vi "main_scan.vi"() -> ()   [LabVIEW 2009]
uses:
  <vilib>/userDefined/High Color/IMAQdx.ctl
  <vilib>/vision/Image Controls.llb/IMAQ Image.ctl
  global_stage_initialised.vi
  <vilib>/vision/driver/IMAQdx.llb/IMAQdx Buffer Number Mode.ctl
  <vilib>/Utility/file.llb/Write To Spreadsheet File (DBL).vi
  <vilib>/vision/driver/NI_Vision_Acquisition_Software.lvlib
  C:/Program Files/National Instruments/LabVIEW 2009/resource/objmgr/imaqdx.rc
panel:
  in  "Max. Spannungsdifferenz":dbl=150.0
  out "Geschätzte Messzeit":string="00:00"
  out "Start time [ms]":timestamp
  out "2D-Intensitätsverteilung (MCP)":dbl[][](graph)
  in  "# Photosignale":i32
  in  "Achs-ID":i32
  in  "Spannungskanal":refnum<k21>
  out "x-U-Scan läuft":bool
  out "Spannungsscan läuft":bool
  out "LAPD Spannung (V)":dbl format="%#.3g"
  out "Summierte Helligkeit (a.u.)":u64
  out "# Messschritte":i32
  out "Aktueller Messschritt":i32
  in  "LAPD-Daten speichern":bool
  in  "Summierte Helligkeit speichern":bool
  in  "Einzelbilder speichern":bool
  in  "Gemittelte Bilder speichern":bool
  in  "# Bilder/Messschritt":i32=1
  in  "SN von Rotationsbühne":i32=83831982
  in  "Wellenplatte [°]":refnum<k7>(container)
  out "Wellenplatte":bool
  in  "Waveplate ON/OFF":bool
  in  "Registerkarte":T1(tab)=enum."x-U-Scan"
  out "Aktuelle xyz-Position [mm]":dbl[](array[numeric]) format="%.5g"
  in  "Rasterweite [µm]":dbl[](array[numeric])
  in  "# Rasterschritte":i32[](array[numeric])=[1, 1, 1] min=1 step=1
  in  "Rasterung ON/OFF":bool
  out "Start xyz-Position [mm]":dbl[](array[numeric]) format="%.5g"
  in  "Rasterart":T2(ring)=enum."2D-Scan(xy)"
  out "Rasterschritt [µm]":dbl[](array[numeric])
  out "2D-Intensitätsverteilung (LAPD)":dbl[][](graph)
  out "Spannungsstart [V]":dbl[](array[numeric])
  out "TIP/SUP":string[](array[string])=["Tip", "Suppressor"]
  out "Spannungsschritt [V]":dbl[](array[numeric]) format="%.1g"
  out "Aktuelle Spannung [V]":dbl[](array[numeric]) format="%.1f"
  in  "# Spannungsschritte":i32[](array[numeric])
  in  "Spannungsweite [V]":dbl[](array[numeric])
  in  "Spannungsscan ON/OFF":bool
  out "x-U-Scan Spannungsstart [V]":dbl
  out "x-U-Scan Spannungsschritt [V]":dbl
  out "x-U-Scan aktuelle Spannung [V]":dbl
  in  "# x-U-Scan Spannungsschritte":i32
  in  "x-U-Scan Spannungsweite [V]":dbl
  in  "Raum-Koordinate":enum16{"x-Achse", "y-Achse", "z-Achse"}(ring)
  in  "Spannungs-Koordinate":enum16{"Tip-Spannung", "Suppressor-Spannung"}(ring)=2
  in  "x-U-Scan ON/OFF":bool
  in  "x-U-Scan Rasterweite [µm]":dbl
  in  "# x-U-Scan Rasterschritte":i32
  out "x-U-Scan Startposition [mm]":dbl format="%.4g"
  out "x-U-Scan aktuelle Position [mm]":dbl format="%.4g"
  out "x-U-Scan Rasterschritt [µm]":dbl
  in  "Sequenz Ordner":string="Referenzbilder"
  in  "Sequenzaufnahme ON":bool
  in  "MCP-Spannung [V]":dbl=1400.0
  in  "P-Schirm-Spannung [V]":dbl=4400.0
  in  "Proben-ID":string="140528_06"
  out "Messlogbuch":path
  out "Gemitteltes Bild":u64[][](array[numeric])
  in  "Polarisation [°]":dbl=90.0
  out "Current y step":i32
  out "Current x step":i32
  out "Current z step":i32
  out "Scanschleifenzähler":i32
  out "Kameraschleifenzähler":i32
  out "Steuerschleifenzähler":i32
  out "Bühne":bool
  in  "HV ON/OFF":bool
  out "HV-Steuerung":bool
  in  "Suppressor-Spannung [V]":dbl min=0.0 max=1000.0 step=1.0 format="%.1p"
  in  "Tip-Spannung [V]":dbl min=0.0 max=800.0 step=1.0 format="%.1p"
  in  "Leistung (iK) [mW]":dbl format="%.1g"
  in  "LAPD-Kanal (Meilhaus)":u32=1 max=31
  out "Save folder":string
  out "Buffer Number":u64
  out "ROI table":string[](array[string])=["Breite [px]", "Höhe [px]", "X-Offset [px]", "Y-Offset [px]"]
  in  "Vollbild":bool
  out "Frame Rate (FPS)":dbl format="%#_3g"
  in  "Buffer Interval":u32=1
  out "Ereignis: FrameDone?":refnum<event-registration>
  out "Image Display":T3(plugin-control)
  in  "ROI":i32[](array[numeric])=[640, 480, 0, 0]
  in  "Shutter time (ms)":u16(ring)=3 items=["1000", "500", "200", "100", "50", "20", "10"]
  out "Buffer Overrun":bool
  out "Image Memory":T3
  out "Kamera":bool
  in  "Kamera ON/OFF":bool
  in  "Detektionskamera":T4="cam0"
  out "Day folder":string
  in  "Root folder":string="E:\\GIPES\\Messungen\\"
  out "z-Achse":i32=3
  out "y-Achse":i32=2
  out "x-Achse":i32=1
  out "Event: Rasterung gestartet?":refnum<user-event>
  out "Fehler (Ausgang)":errorcluster
  in  "Programm beenden":bool
  out "Rasterung läuft":bool
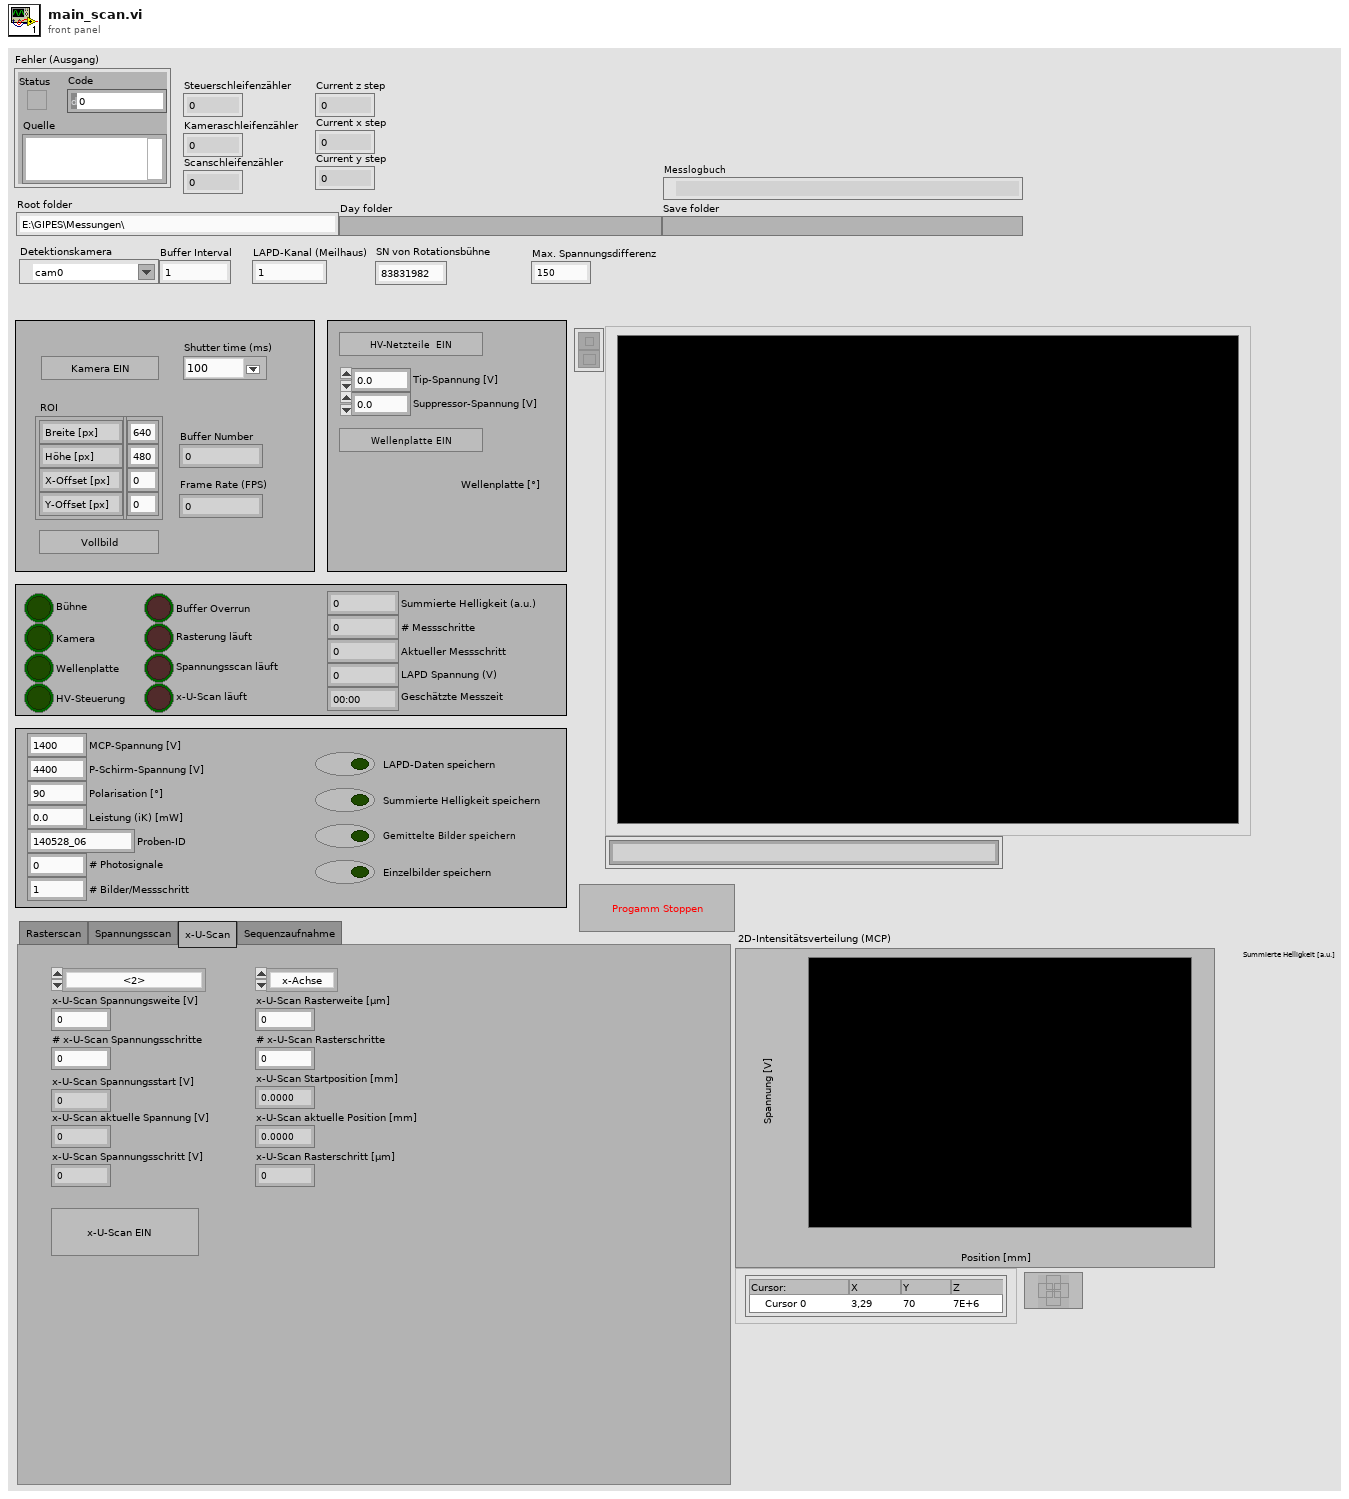
[diagram p1: front panel]
types:
  T1 = enum32{"Rasterscan", "Spannungsscan", "x-U-Scan", "Sequenzaufnahme"}
  T2 = enum16{"Linescan(x)", "Linescan(z)", "2D-Scan(xy)", "2D-Scan(yz)"}
  T3 = typedef "IMAQ Image.ctl" = refnum<image>
  T4 = typedef "IMAQdx.ctl" = refnum<k21>
  T5 = enum32{"Bad", "Idle", "Run top level", "Running"}
  T6 = typedef "NI_Vision_Acquisition_Software.lvlib/IMAQdx Buffer Number Mode.ctl" = enum32{"Next", "Last", "Buffer Number"}
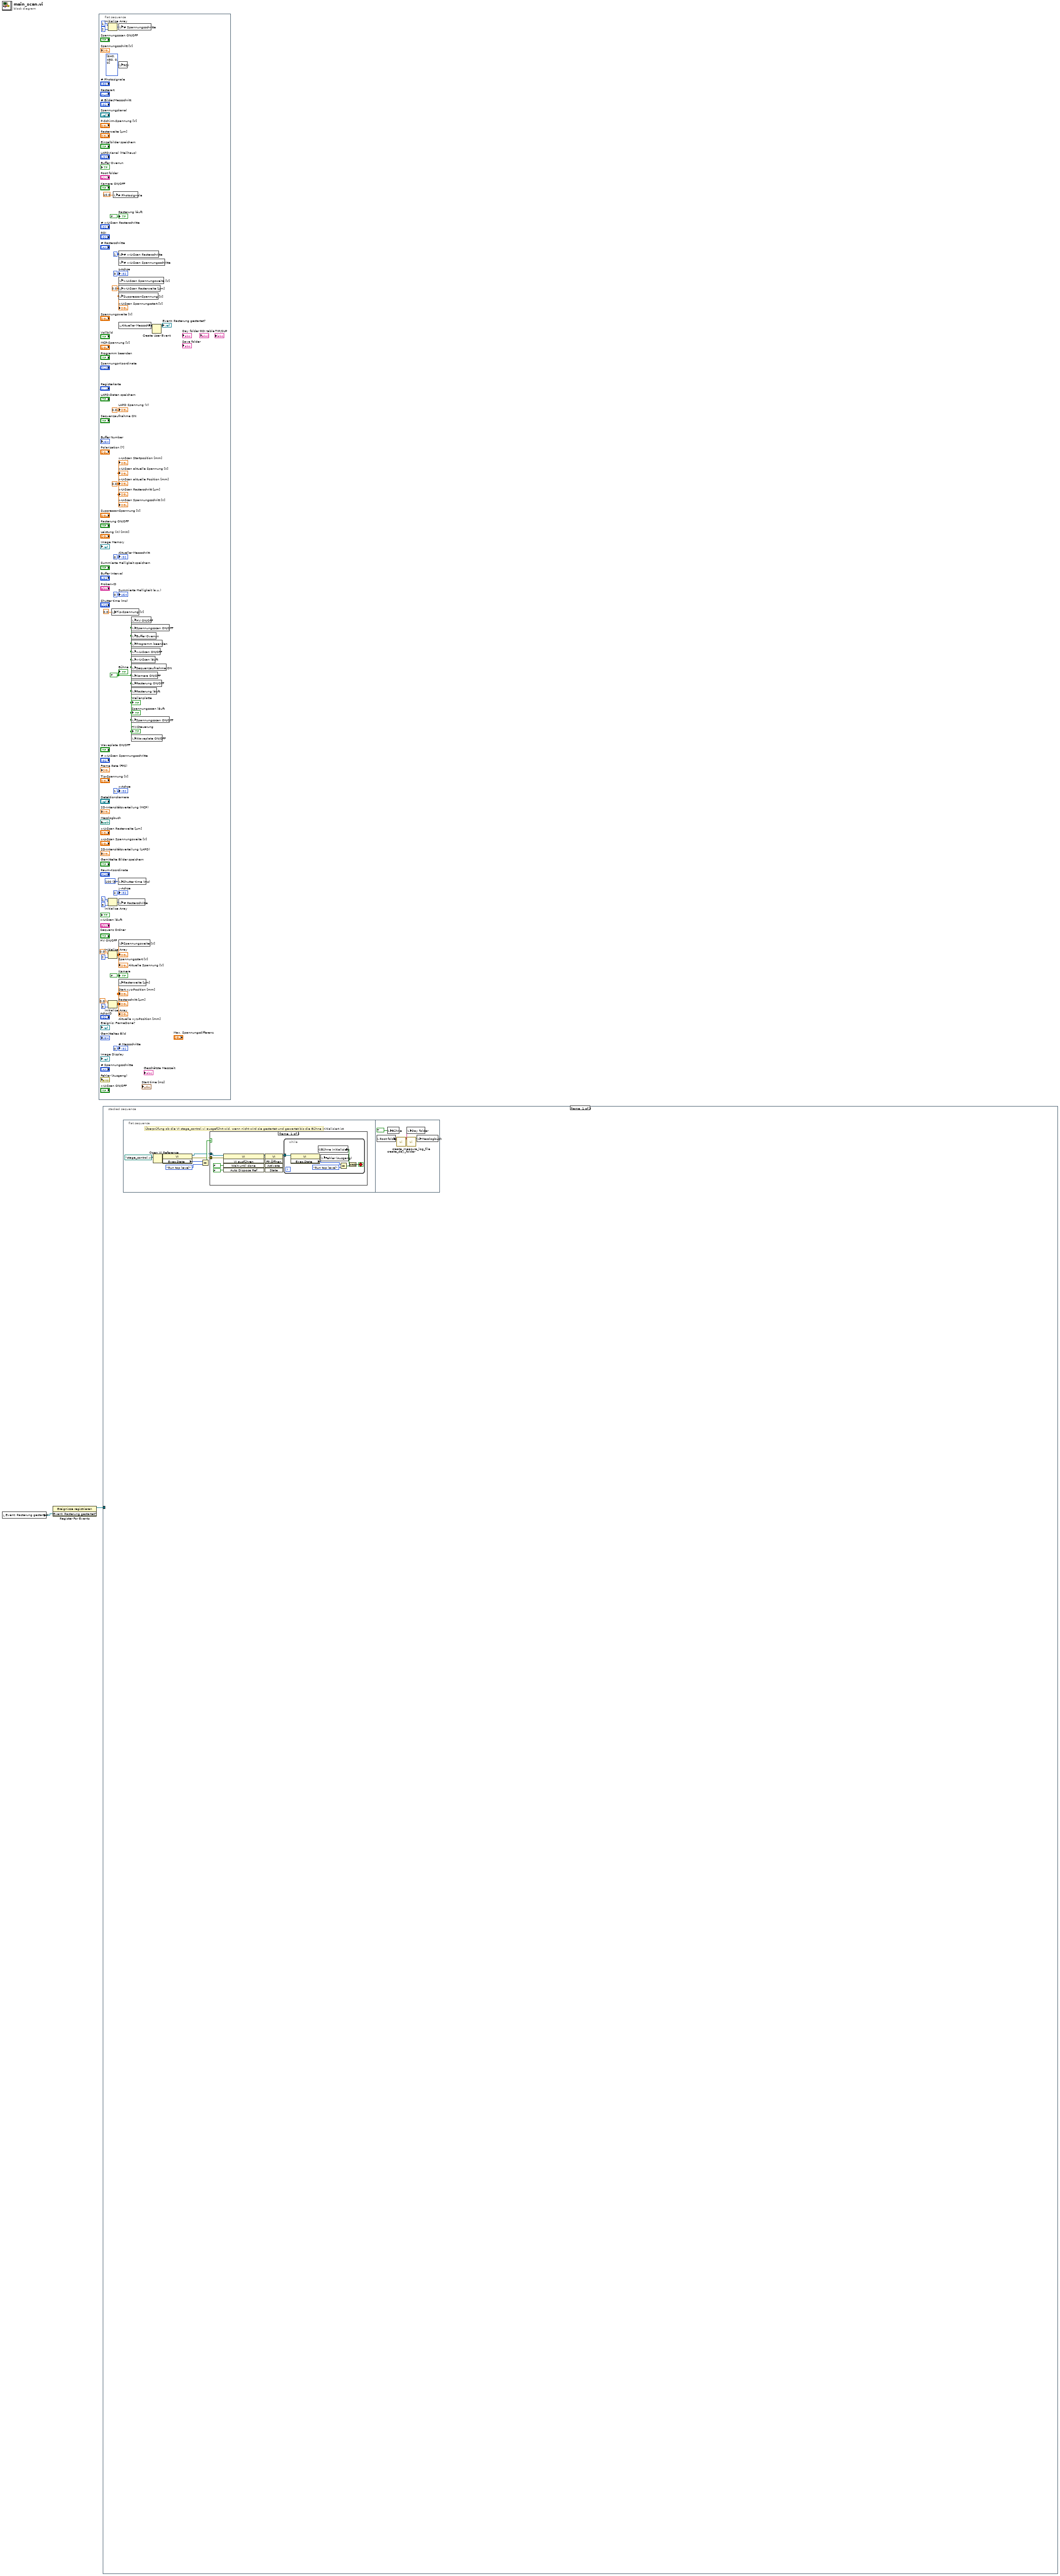
[diagram p0: block diagram]
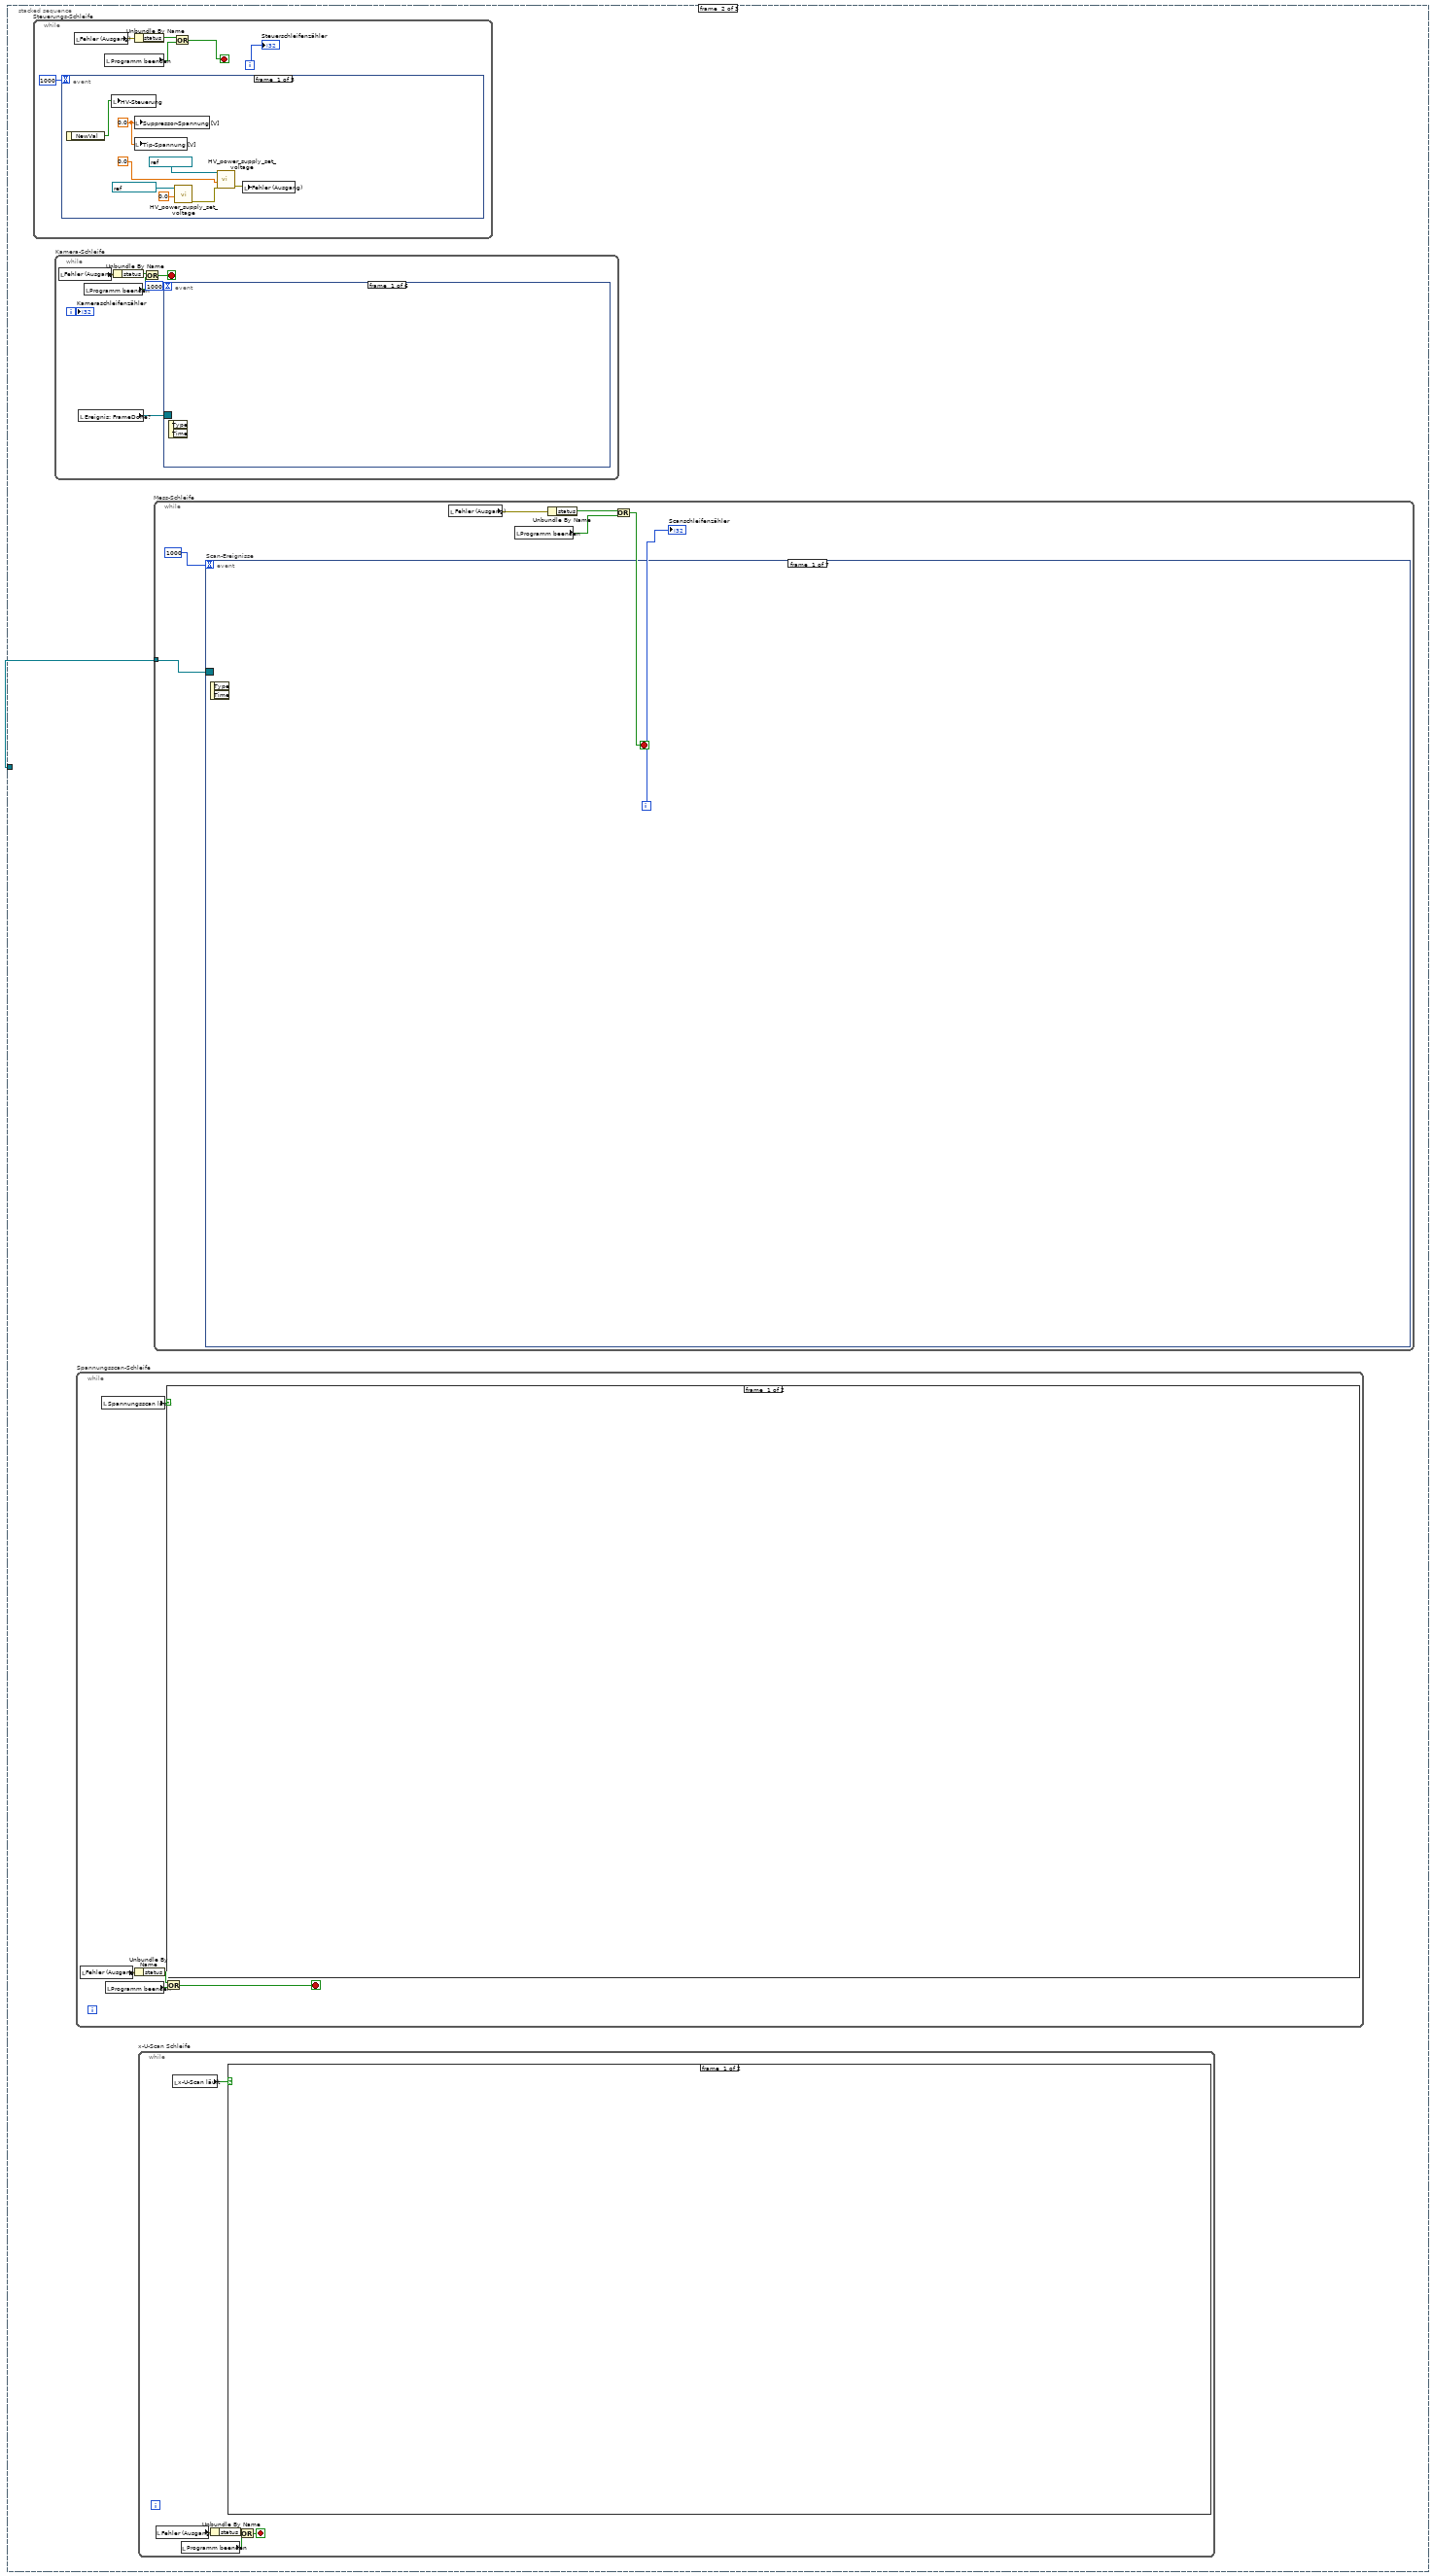
[diagram p3: hidden frame]
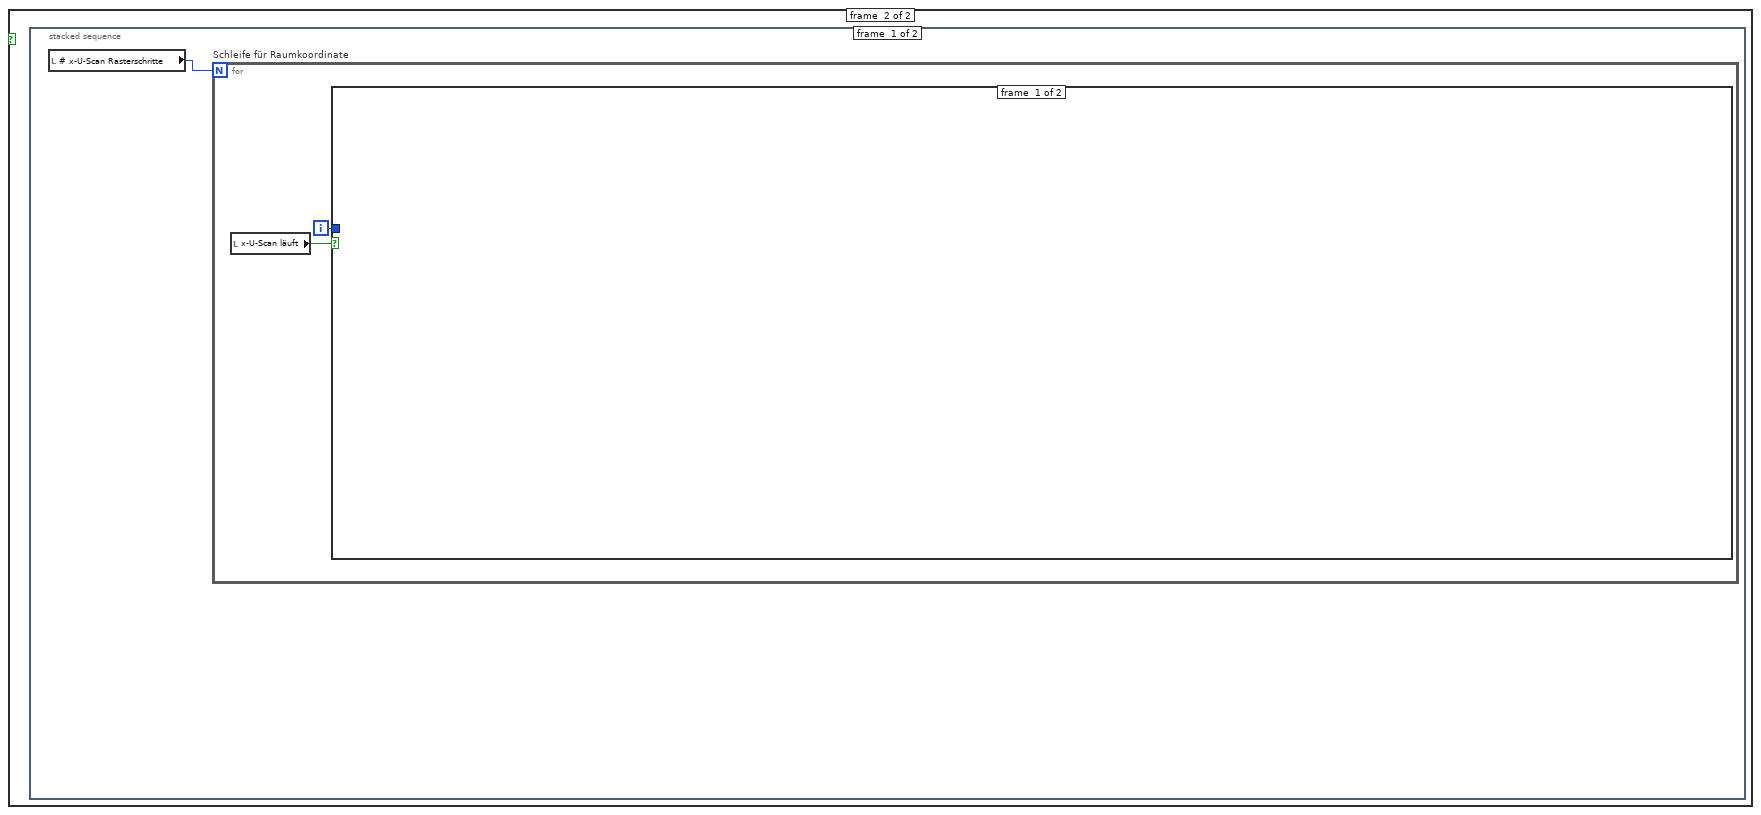
[diagram p4: hidden frame]
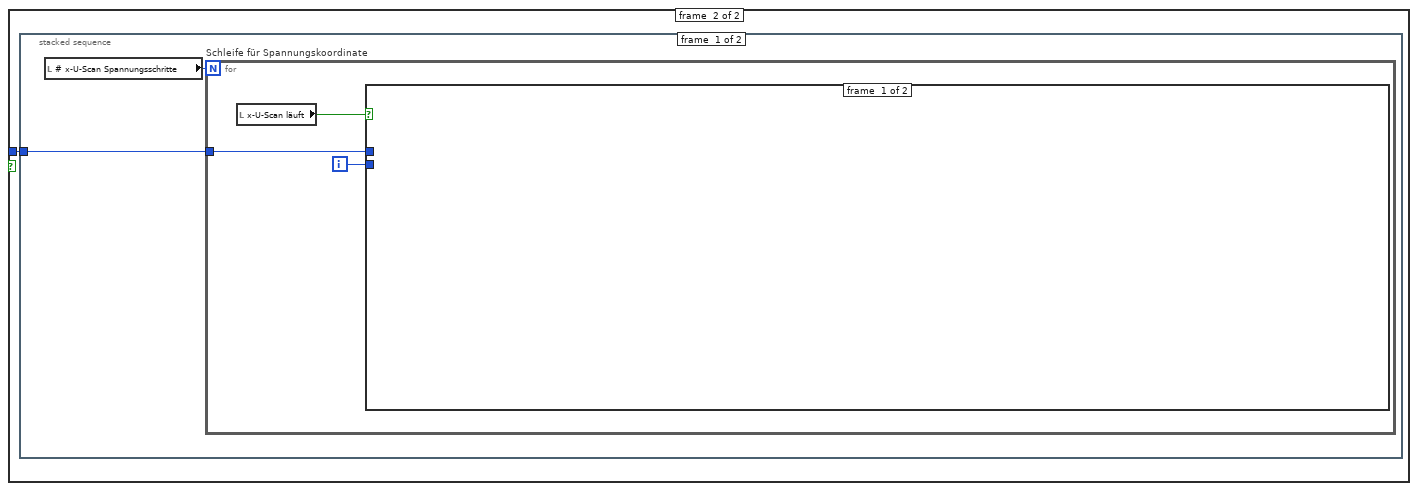
[diagram p5: hidden frame]
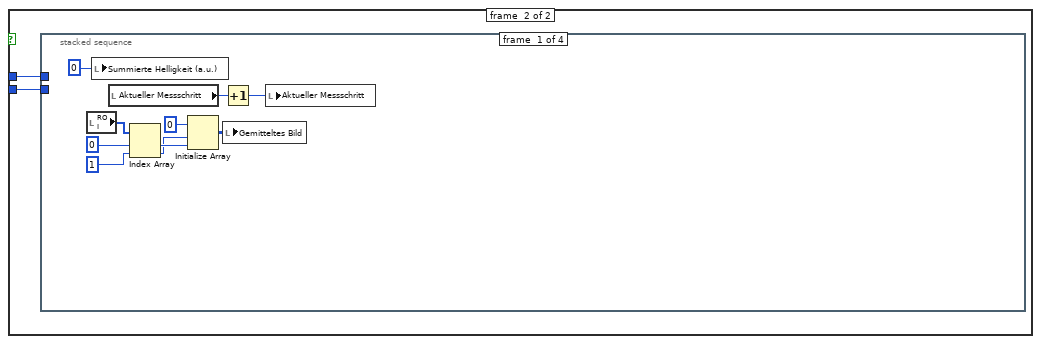
[diagram p6: hidden frame]
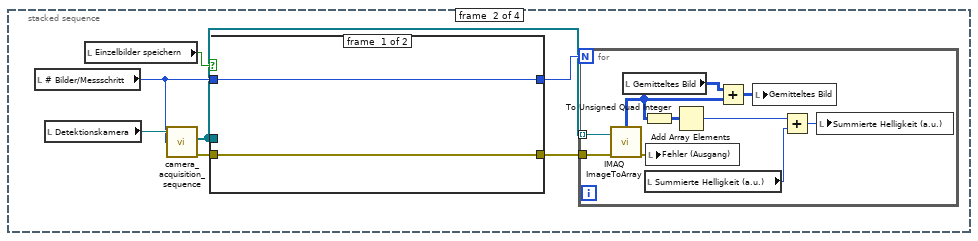
[diagram p7: hidden frame]
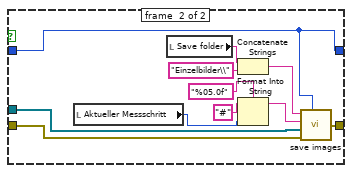
[diagram p8: hidden frame]
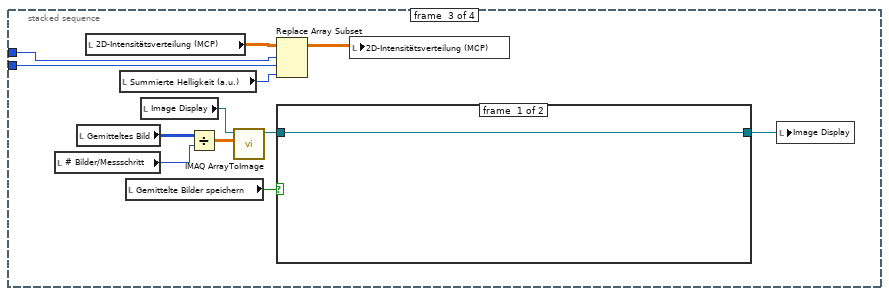
[diagram p9: hidden frame]
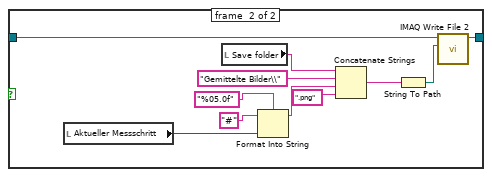
[diagram p10: hidden frame]
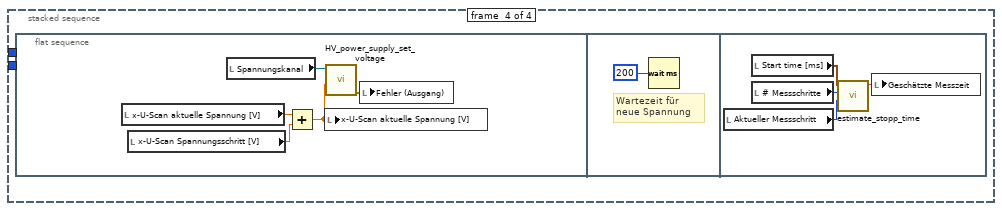
[diagram p11: hidden frame]
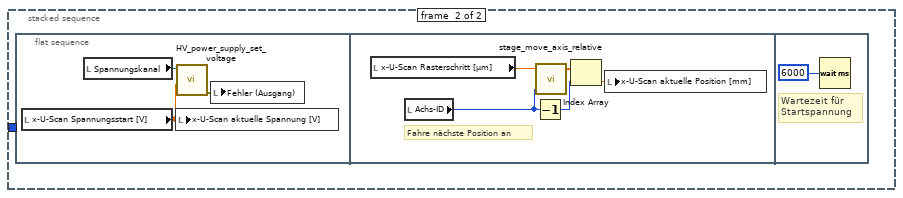
[diagram p12: hidden frame]
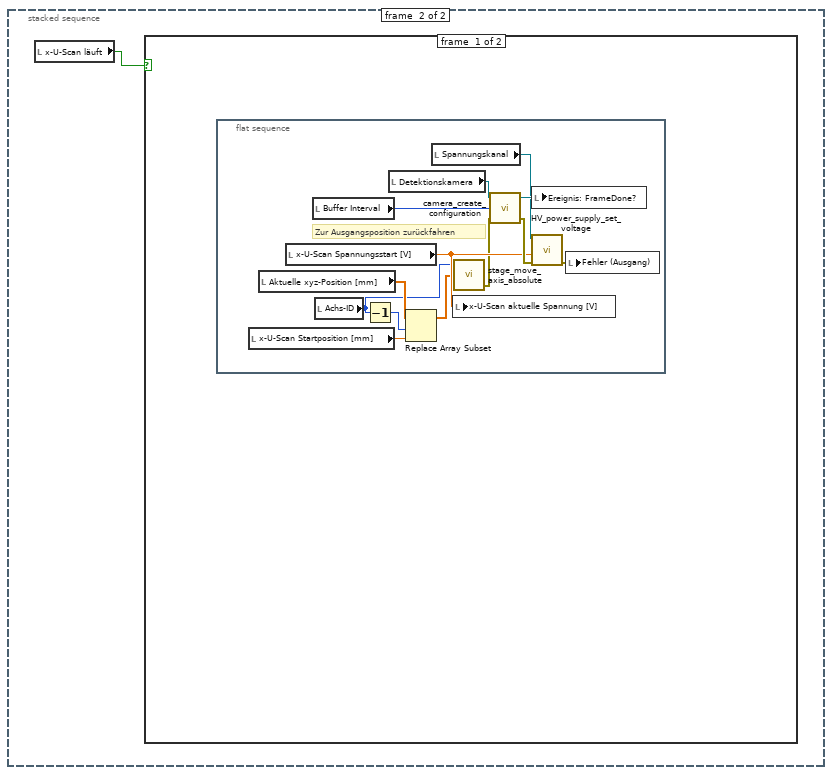
[diagram p13: hidden frame]
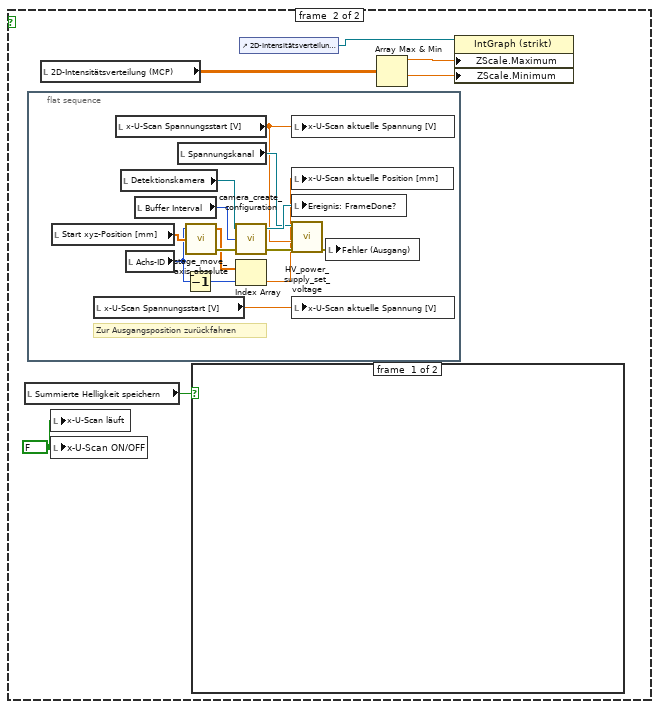
[diagram p14: hidden frame]
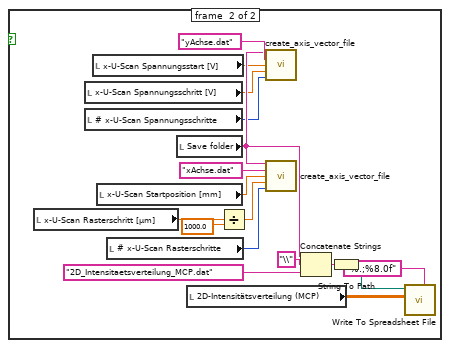
[diagram p15: hidden frame]
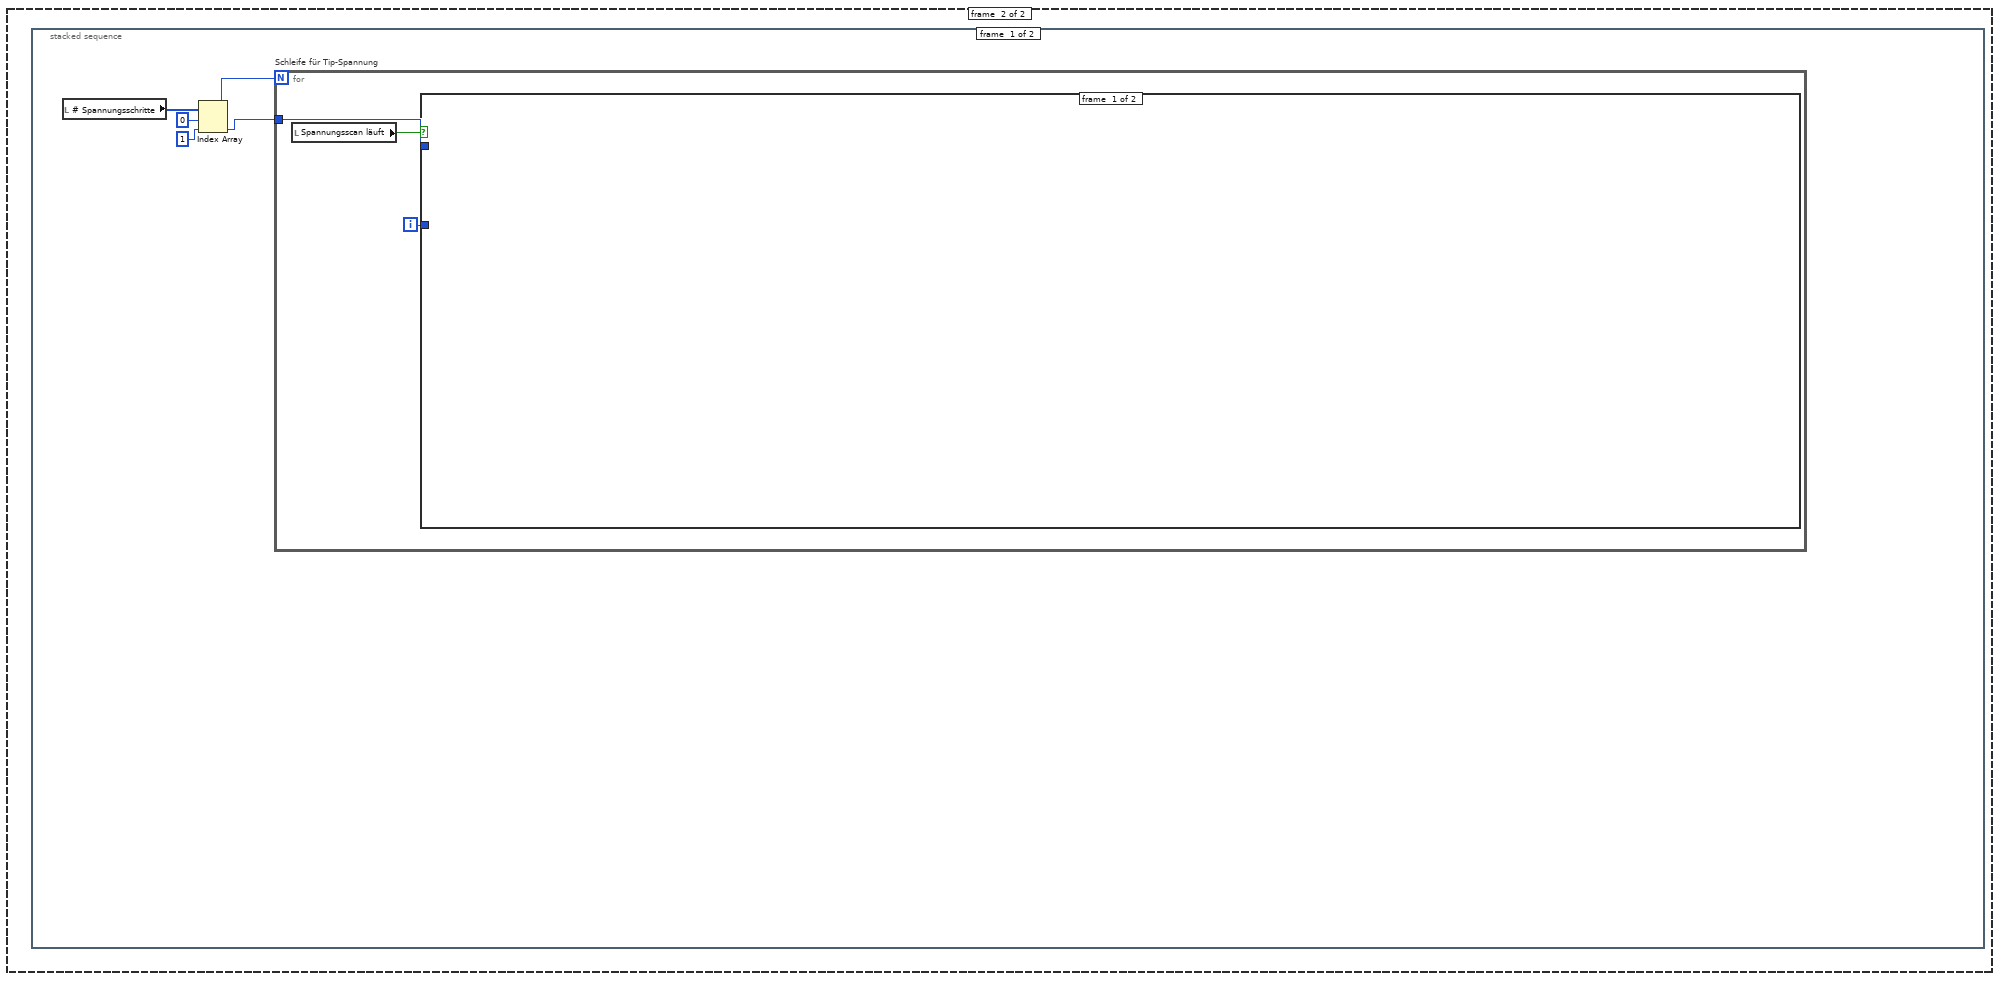
[diagram p16: hidden frame]
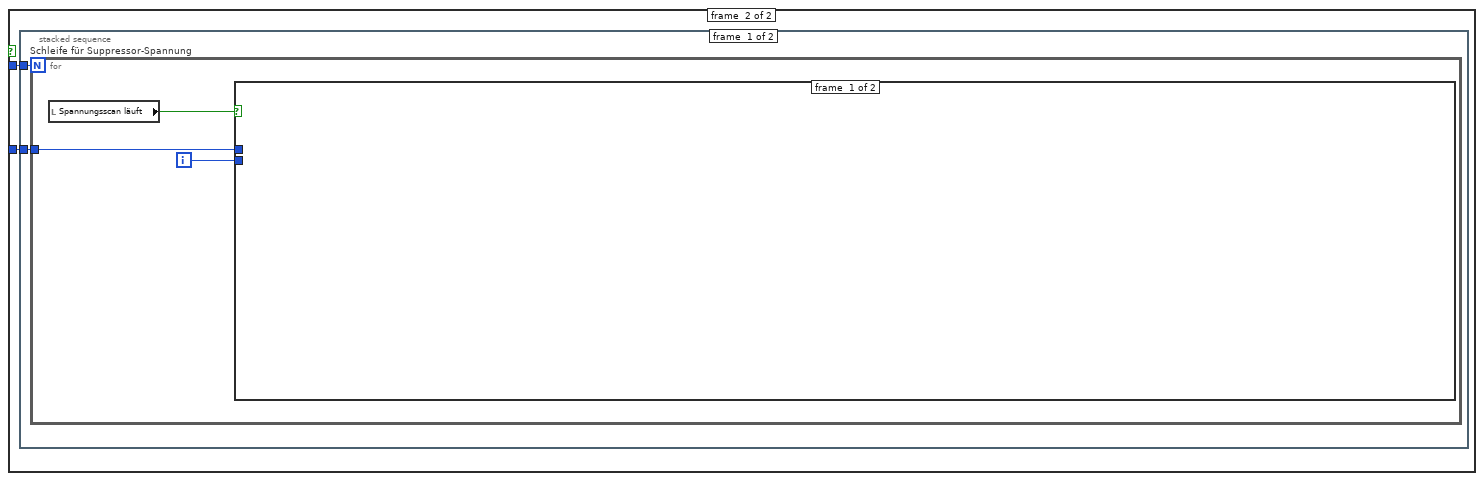
[diagram p17: hidden frame]
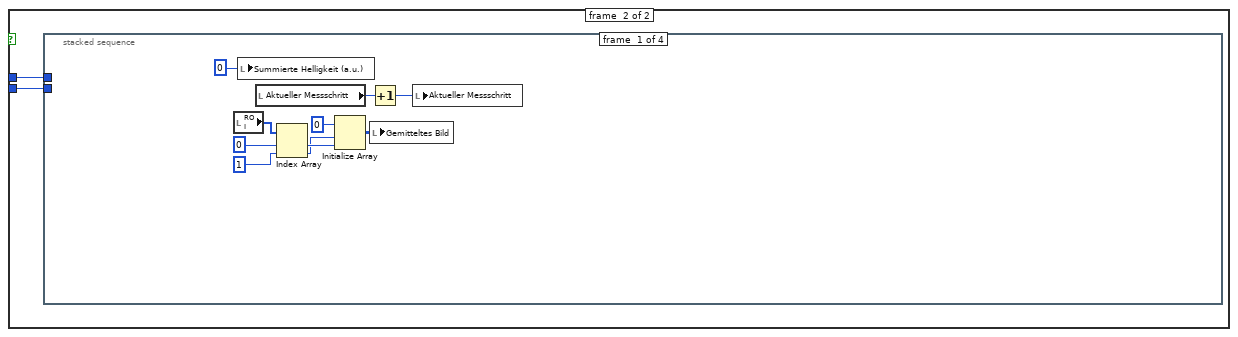
[diagram p18: hidden frame]
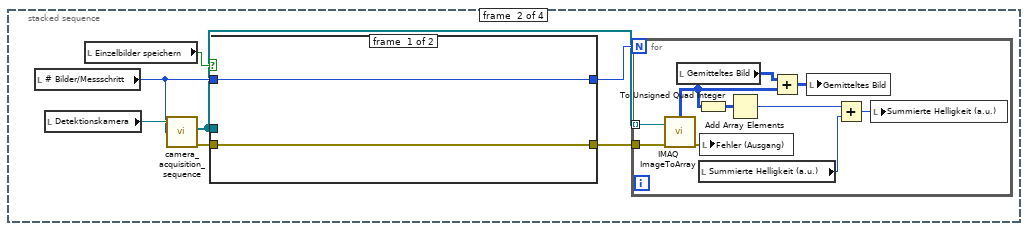
[diagram p19: hidden frame]
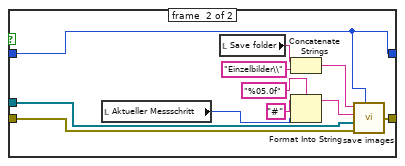
[diagram p20: hidden frame]
diagram:
  n1 = local read "Event: Rasterung gestartet?"() -> (w2:refnum<user-event>)
  n2 = register-events(w2) -> (reference out=w1:refnum<event-registration>)  [unwired: 2 in, 1 out]
  n3 = flat-sequence {
    frame #0 {
      w6 = 1 ("# x-U-Scan Spannungsschritte")
      w7 = 0.0 ("Aktuelle x-Position [mm]")
      w3 = 0.0 ("Suppressor-Spannung [V]")
      w20 = u16 3 items=["1000", "500", "200", "100", "50", "20", "10"] ("Shutter time (ms)")
      w5 = FALSE ("Scanstart")
      n4 = Initialize Array(1 ("Element"), 2 ("Dimension")) -> (w8:i32[])
      n5 = Initialize Array(1 ("Dimension"), 3 ("Dimension")) -> (w32:i32[])
      n6 = Initialize Array(0.0 ("Element"), 2 ("Dimension")) -> (w4:dbl[])
      "Aktuelle Spannung [V]" <- w4
      "Spannungsstart [V]" <- w4
      n7 = Initialize Array(0.0 ("Element"), 3 ("Dimension")) -> (w14:dbl[])
      "Aktuelle xyz-Position [mm]" <- w14
      "Start xyz-Position [mm]" <- w14
      "Rasterschritt [µm]" <- w14
      n8 = local write "Tip-Spannung [V]"(0.0 ("Tip-Spannung [V]")) -> ()
      n9 = local write "# Photosignale"(10.0 ("Anzahl Mittelungen")) -> ()
      n10 = local write "Shutter time (ms)"(w20) -> ()
      n11 = local write "# Spannungsschritte"(w8) -> ()
      n12 = local write "ROI"(i32[] [640, 480, 0, 0] ("Region of Interest (px)")) -> ()
      n13 = local write "# x-U-Scan Rasterschritte"(w6) -> ()
      n14 = local write "# x-U-Scan Spannungsschritte"(w6) -> ()
      n15 = local write "x-U-Scan Spannungsweite [V]"(w3) -> ()
      n16 = local write "x-U-Scan Rasterweite [µm]"(w3) -> ()
      n17 = local write "Suppressor-Spannung [V]"(w3) -> ()
      n18 = local read "Aktueller Messschritt"() -> (w25:i32)
      n19 = local write "# Rasterschritte"(w32) -> ()
      n20 = local write "Spannungsweite [V]"(w4) -> ()
      n21 = local write "Rasterweite [µm]"(w14) -> ()
      n22 = local write "HV ON/OFF"(w5) -> ()
      n23 = local write "Spannungsscan ON/OFF"(w5) -> ()
      n24 = local write "Buffer Overrun"(w5) -> ()
      n25 = local write "Programm beenden"(w5) -> ()
      n26 = local write "x-U-Scan ON/OFF"(w5) -> ()
      n27 = local write "x-U-Scan läuft"(w5) -> ()
      n28 = local write "Sequenzaufnahme ON"(w5) -> ()
      n29 = local write "Kamera ON/OFF"(w5) -> ()
      n30 = local write "Rasterung ON/OFF"(w5) -> ()
      n31 = local write "Rasterung läuft"(w5) -> ()
      n32 = local write "Spannungsscan ON/OFF"(w5) -> ()
      n33 = local write "Waveplate ON/OFF"(w5) -> ()
      n34 = Create User Event(user event datatype=w25) -> (user event=→"Event: Rasterung gestartet?":refnum<user-event>)  [unwired: 1 in, 1 out]
      "Rasterung läuft" <- FALSE ("Scan aktiv")
      "# Messschritte" <- 0 ("# Messschritte")
      "Aktueller Messschritt" <- 0 ("Aktueller Messschritt")
      "x-Achse" <- 1 ("x-Achse")
      "y-Achse" <- 2 ("y-Achse")
      "z-Achse" <- 3 ("z-Achse")
      "Summierte Helligkeit (a.u.)" <- i64 0 ("Numerisches Element")
      "LAPD Spannung (V)" <- 0.0 ("Transmittierte Intensität (a.u.)")
      "Bühne" <- w5
      "Wellenplatte" <- w5
      "Kamera" <- FALSE ("Camera eingeschaltet")
      "HV-Steuerung" <- w5
      "Spannungsscan läuft" <- w5
      "x-U-Scan aktuelle Position [mm]" <- w7
      "x-U-Scan Rasterschritt [µm]" <- w7
      "x-U-Scan aktuelle Spannung [V]" <- w7
      "x-U-Scan Spannungsschritt [V]" <- w7
      "x-U-Scan Startposition [mm]" <- w7
      "x-U-Scan Spannungsstart [V]" <- w3
    }
  }
  n35 = stacked-sequence {
    tunnel: w1 -> [_ w58 _]
    frame #0 {
      n36 = flat-sequence {
        frame #0 {
          # "Überprüfung ob die VI stage_control.vi ausgeführt wid, wenn nicht wird sie gestartet und gewartet bis die Bühne initialisiert ist"
          n37 = Open VI Reference(vi path=path "stage_control.vi" ("VI-Pfad")) -> (vi reference=w36:refnum<vi>)  [unwired: 5 in, 1 out]
          n38 = property class="VI"(reference=w36) -> (reference out=w35:refnum<vi>, error out=w34:errorcluster, "Exec.State"=w39:T5)  [unwired: 1 in]
          n39 = Equal?(x=w39, y=T5."Run top level") -> (x = y?=w37:bool)
          n40 = case shown="False" w37 {
            tunnel: w35 -> [w46 _]
            tunnel: w34 -> [w45 _]
            frame #0 {
              n41 = invoke class="VI" method="VI ausführen"(reference=w46, error in=w45, "Wait until done"=FALSE ("Warten bis beendet"), "Auto Dispose Ref"=FALSE ("Referenz automatisch schließen")) -> (reference out=w42:refnum<vi>)  [unwired: 1 in, 4 out]
              n42 = invoke class="VI" method="FP.Öffnen"(reference=w42) -> (reference out=w41:refnum<vi>)  [unwired: 4 in, 4 out]
              n43 = while {
                tunnel: w41 -> [w53]
                stop <- w48 stop-if-true
                n44 = property class="VI"(reference=w53) -> (error out=w52:errorcluster, "Exec.State"=w51:T5)  [unwired: 1 in, 1 out]
                n45 = global read "global_stage_initialised.vi" "Bühne initialisiert"() -> (w47:bool)
                n46 = local write "Fehler (Ausgang)"(w52) -> ()
                n47 = Equal?(x=w51, y=T5."Run top level") -> (x = y?=w49:bool)
                n48 = And(x=w47, y=w49) -> (x .and. y?=w48:bool)
              }
            }
            frame #1 {
            }
          }
        }
        frame #1 {
          n49 = local read "Root folder"() -> (w57:string)
          n50 = local write "Bühne"(TRUE ("Bühne bereit")) -> ()
          n51 = call "create_day_folder.vi"("Root folder"=w57) -> ("Day Folder"=w55:string)  [unwired: 9 in, 1 out]
          n52 = local write "Day folder"(w55) -> ()
          n53 = call "create_measure_log_file.vi"("Tagesordner"=w55) -> ("Messlogbuch"=w54:path)  [unwired: 9 in]
          n54 = local write "Messlogbuch"(w54) -> ()
        }
      }
    }
    frame #1 {
      n55 = while "Steuerungs-Schleife" {
        i -> [w387]
        stop <- w386 stop-if-true
        n56 = event shown="[2] \"Tip-Spannung [V]\": Wertänderung" {
          selector: _ -> [_ _ _ _ _]
          dyn-events: _ -> [_ _ _ _ _]
          timeout: 1000 -> [_ _ _ _ _]
          event #0 {
            w392 = 0.0 ("Suppressor-Spannung [V]")
            n57 = event-data() -> ("NewVal"=w393:bool)  [unwired: 1 in]
            n58 = local write "HV-Steuerung"(w393) -> ()
            n59 = local write "Suppressor-Spannung [V]"(w392) -> ()
            n60 = local write "Tip-Spannung [V]"(w392) -> ()
            n61 = call "HV_power_supply_set_voltage.vi"("Desired output voltage in V (HV power supply)"=0.0, "Channel of HV power supply"=refnum<k21> "Dev0/Ao0") -> ("error out"=w395:errorcluster)  [unwired: 8 in]
            n62 = call "HV_power_supply_set_voltage.vi"("error in"=w395, "Desired output voltage in V (HV power supply)"=0.0, "Channel of HV power supply"=refnum<k21> "Dev0/Ao1") -> ("error out"=w394:errorcluster)  [unwired: 7 in]
            n63 = local write "Fehler (Ausgang)"(w394) -> ()
          }
          event #1 {
            n64 = event-data() -> ("NewVal"=w400:bool)  [unwired: 1 in]
            n65 = case shown="True" w400 {
              frame #0 {
                n66 = local read "Wellenplatte [°]"() -> (w403:refnum<k7>)
                n67 = invoke class="MG17Motor" method="StopCtrl"(reference=w403) -> (error out=w402:errorcluster)  [unwired: 2 in, 2 out]
                n68 = Unbundle By Name(w402) -> ("status"=w401:bool)
                n69 = local write "Wellenplatte"(w401) -> ()
              }
              frame #1 {
                n70 = property class="MG17Motor"(reference="Wellenplatte [°]", "HWSerialNum"="SN von Rotationsbühne") -> (reference out=w410:refnum<k7>, error out=w409:errorcluster)  [unwired: 1 in]
                n71 = invoke class="MG17Motor" method="StartCtrl"(reference=w410, error in=w409) -> (error out=w408:errorcluster)  [unwired: 1 in, 2 out]
                n72 = local write "Fehler (Ausgang)"(w408) -> ()
                n73 = Unbundle By Name(w408) -> ("status"=w407:bool)
                n74 = Not(x=w407) -> (.not. x?=w406:bool)
                n75 = local write "Wellenplatte"(w406) -> ()
              }
            }
          }
          event #2 {
            n76 = event-data() -> ("OldVal"=w411:dbl, "NewVal"=w417:dbl)  [unwired: 1 in]
            n77 = local read "Suppressor-Spannung [V]"() -> (w416:dbl)
            n78 = local read "Max. Spannungsdifferenz"() -> (w414:dbl)
            n79 = local read "HV-Steuerung"() -> (w412:bool)
            n80 = Subtract(x=w417, y=w416) -> (x-y=w415:dbl)
            n81 = Less Or Equal?(x=w415, y=w414) -> (x <= y?=w413:bool)
            n82 = case shown="True" w412 {
              tunnel: w413 -> [_ w419]
              tunnel: w411 -> [_ w418]
              frame #0 {
              }
              frame #1 {
                n83 = case shown="True" w419 {
                  tunnel: w418 -> [w420 _]
                  frame #0 {
                    n84 = local write "Tip-Spannung [V]"(w420) -> ()
                  }
                  frame #1 {
                    n85 = local read "Tip-Spannung [V]"() -> (w421:dbl)
                    n86 = call "HV_power_supply_set_voltage.vi"("Desired output voltage in V (HV power supply)"=w421, "Channel of HV power supply"=refnum<k21> "Dev0/Ao1") -> ("error out"=w422:errorcluster)  [unwired: 8 in]
                    n87 = local write "Fehler (Ausgang)"(w422) -> ()
                  }
                }
              }
            }
          }
          event #3 {
            n88 = event-data() -> ("OldVal"=w424:dbl, "NewVal"=w426:dbl)  [unwired: 1 in]
            n89 = local read "Max. Spannungsdifferenz"() -> (w427:dbl)
            n90 = local read "Tip-Spannung [V]"() -> (w425:dbl)
            n91 = local read "HV-Steuerung"() -> (w430:bool)
            n92 = Subtract(x=w425, y=w426) -> (x-y=w429:dbl)
            n93 = Less Or Equal?(x=w429, y=w427) -> (x <= y?=w428:bool)
            n94 = case shown="True" w430 {
              tunnel: w428 -> [_ w432]
              tunnel: w424 -> [_ w431]
              frame #0 {
              }
              frame #1 {
                n95 = case shown="True" w432 {
                  tunnel: w431 -> [w433 _]
                  frame #0 {
                    n96 = local write "Suppressor-Spannung [V]"(w433) -> ()
                  }
                  frame #1 {
                    n97 = local read "Suppressor-Spannung [V]"() -> (w434:dbl)
                    n98 = call "HV_power_supply_set_voltage.vi"("Desired output voltage in V (HV power supply)"=w434, "Channel of HV power supply"=refnum<k21> "Dev0/Ao0") -> ("error out"=w435:errorcluster)  [unwired: 8 in]
                    n99 = local write "Fehler (Ausgang)"(w435) -> ()
                  }
                }
              }
            }
          }
          event #4 {
            n100 = event-data() -> ()  [unwired: 1 in, 2 out]
          }
        }
        n101 = local read "Fehler (Ausgang)"() -> (w391:errorcluster)
        n102 = local read "Programm beenden"() -> (w390:bool)
        n103 = Unbundle By Name(w391) -> ("status"=w389:bool)
        n104 = Or(x=w389, y=w390) -> (x .or. y?=w386:bool)
        "Steuerschleifenzähler" <- w387
      }
      n105 = while "Kamera-Schleife" {
        i -> [w1158]
        stop <- w1159 stop-if-true
        n106 = local read "Fehler (Ausgang)"() -> (w1160:errorcluster)
        n107 = local read "Ereignis: FrameDone?"() -> (w1163:refnum<event-registration>)
        n108 = local read "Programm beenden"() -> (w1162:bool)
        n109 = Unbundle By Name(w1160) -> ("status"=w1161:bool)
        n110 = Or(x=w1161, y=w1162) -> (x .or. y?=w1159:bool)
        n111 = event "Kamera-Ereignisse" shown="[1] \"Kamera ON/OFF\": Wertänderung" {
          selector: w1163 -> [_ _ _ _ _ _]
          dyn-events: _ -> [_ _ _ _ _ _]
          timeout: 1000 -> [_ _ _ _ _ _]
          event #0 {
            n112 = event-data() -> ()  [unwired: 1 in, 2 out]
          }
          event #1 {
            n113 = event-data() -> ()  [unwired: 1 in, 4 out]
            n114 = local read "Detektionskamera"() -> (w1166:T4)
            n115 = local read "Kamera ON/OFF"() -> (w1167:bool)
            n116 = case shown="True" w1167 {
              tunnel: w1166 -> [w1168 w1173]
              tunnel: [w1171 w1174] -> w1165
              frame #0 {
                n117 = local read "Image Memory"() -> (w1169:T3)
                n118 = call "camera_release configuration_stop.vi"("Image Memory"=w1169, "Detektionskamera"=w1168) -> ("error out"=w1171:errorcluster, "status"=w1170:bool)
                n119 = local write "Kamera"(w1170) -> ()
              }
              frame #1 {
                n120 = local read "Buffer Interval"() -> (w1172:u32)
                n121 = call "camera_acquisition_continously.vi"("BufferInterval"=w1172, "Detektionskamera"=w1173) -> ("error out"=w1174:errorcluster, "Ereignis: FrameDone?"=w1175:refnum<event-registration>, "Image Memory"=w1176:T3, "Detektionskamera"=w1177:T4, "Kamera eingeschaltet?"=w1178:bool)
                n122 = local write "Kamera"(w1178) -> ()
                n123 = local write "Detektionskamera"(w1177) -> ()
                n124 = local write "Image Memory"(w1176) -> ()
                n125 = local write "Ereignis: FrameDone?"(w1175) -> ()
              }
            }
            n126 = local write "Fehler (Ausgang)"(w1165) -> ()
          }
          event #2 {
            w1191 = IMAQdx_Buffer_Number_Mode."Buffer Number"  # Buffer Number Mode
            n127 = event-data() -> ("ActualBufferNumber"=w1185:u32)  [unwired: 1 in]
            n128 = local read "Detektionskamera"() -> (w1190:T4)
            n129 = local read "Image Memory"() -> (w1189:T3)
            n130 = call <vilib>:"IMAQdx Get Image.vi"("Buffer Number Mode (Next)"=w1191, "Buffer Number In"=w1185, "Image In"=w1189, "Session In"=w1190) -> ("error out"=w1183:errorcluster, "Buffer Number Out"=w1186:u32, "Image Out"=w1182:T3, "Session Out"=w1187:T4)  [unwired: 1 in, 3 out]
            n131 = Not Equal?(x=w1186, y=w1185) -> (x != y?=w1184:bool)
            n132 = local write "Detektionskamera"(w1187) -> ()
            n133 = local write "Image Display"(w1182) -> ()
            n134 = call "IMAQ ImageToArray"("Image"=w1182) -> ("Image Pixels (U8)"=w1181:u8[][])  [unwired: 3 in, 4 out]
            n135 = local write "Image Memory"(w1182) -> ()
            n136 = local write "Buffer Number"(w1186) -> ()
            n137 = call "CalculateFPS.vi"("buffer number"=w1186) -> ("processed FPS"=w1188:dbl)  [unwired: 2 out]
            n138 = local write "Fehler (Ausgang)"(w1183) -> ()
            n139 = To Unsigned Quad Integer(1:w1181) -> (0:w1180:u64[][])
            n140 = local write "Frame Rate (FPS)"(w1188) -> ()
            n141 = local write "Buffer Overrun"(w1184) -> ()
            n142 = Add Array Elements(numeric array=w1180) -> (sum=w1179:u64)
            n143 = local write "Summierte Helligkeit (a.u.)"(w1179) -> ()
          }
          event #3 {
            n144 = event-data() -> ()  [unwired: 1 in, 2 out]
            n145 = local read "Kamera"() -> (w1192:bool)
            n146 = case shown="True" w1192 {
              frame #0 {
              }
              frame #1 {
                n147 = control-ref of="Shutter time (ms)"() -> (w1199:refnum<vi>)
                n148 = property class="Ring (strikt)"(reference=w1199) -> ("RingText.Text"=w1198:string)  [unwired: 1 in, 2 out]
                n149 = local read "Detektionskamera"() -> (w1197:T4)
                n150 = Decimal String To Number(string=w1198) -> (number=w1194:i32)  [unwired: 2 in, 1 out]
                n151 = property class="IMAQdx"(reference=w1197, "ActiveAttribute"="CameraAttributes::Shutter::Value", "ValueDBL"=w1194) -> (reference out=w1196:T4, error out=w1193:errorcluster)  [unwired: 1 in]
                n152 = local write "Detektionskamera"(w1196) -> ()
                n153 = local write "Fehler (Ausgang)"(w1193) -> ()
              }
            }
          }
          event #4 {
            n154 = event-data() -> ()  [unwired: 1 in, 1 out]
            n155 = local read "Kamera"() -> (w1200:bool)
            n156 = case shown="True" w1200 {
              frame #0 {
              }
              frame #1 {
                n157 = local read "Ereignis: FrameDone?"() -> (w1202:refnum<event-registration>)
                n158 = local read "Detektionskamera"() -> (w1206:T4)
                n159 = local read "Buffer Interval"() -> (w1205:u32)
                n160 = local read "ROI"() -> (w1207:i32[])
                n161 = call "camera_change_ROI.vi"("BufferInterval"=w1205, "Region of Interest"=w1207, "Ereignisregistrierung (Referenz) 2"=w1202, "Session In"=w1206) -> ("Fehler (Ausgang)"=w1201:errorcluster, "Ereignisregistrierung (Referenz)"=w1204:refnum<event-registration>, "Session Out"=w1203:T4)  [unwired: 5 in]
                n162 = local write "Detektionskamera"(w1203) -> ()
                n163 = local write "Ereignis: FrameDone?"(w1204) -> ()
                n164 = local write "Fehler (Ausgang)"(w1201) -> ()
              }
            }
          }
          event #5 {
            n165 = event-data() -> ("NewVal"=w1209:bool)  [unwired: 1 in, 1 out]
            n166 = local read "Kamera"() -> (w1210:bool)
            n167 = And(x=w1210, y=w1209) -> (x .and. y?=w1208:bool)
            n168 = case shown="True" w1208 {
              frame #0 {
              }
              frame #1 {
                n169 = local read "Ereignis: FrameDone?"() -> (w1213:refnum<event-registration>)
                n170 = local read "Detektionskamera"() -> (w1217:T4)
                n171 = local read "Buffer Interval"() -> (w1216:u32)
                n172 = call "camera_change_ROI.vi"("BufferInterval"=w1216, "Region of Interest"=i32[] [640, 480, 0, 0] ("Region of Interest (px)"), "Ereignisregistrierung (Referenz) 2"=w1213, "Session In"=w1217) -> ("Fehler (Ausgang)"=w1211:errorcluster, "Ereignisregistrierung (Referenz)"=w1215:refnum<event-registration>, "Session Out"=w1214:T4)  [unwired: 5 in]
                n173 = local write "Detektionskamera"(w1214) -> ()
                n174 = local write "Ereignis: FrameDone?"(w1215) -> ()
                n175 = local write "Fehler (Ausgang)"(w1211) -> ()
              }
            }
          }
        }
        "Kameraschleifenzähler" <- w1158
      }
      n176 = while "Spannungsscan-Schleife" {
        stop <- w210 stop-if-true
        n177 = local read "Fehler (Ausgang)"() -> (w211:errorcluster)
        n178 = local read "Spannungsscan läuft"() -> (w209:bool)
        n179 = local read "Programm beenden"() -> (w213:bool)
        n180 = Unbundle By Name(w211) -> ("status"=w212:bool)
        n181 = Or(x=w212, y=w213) -> (x .or. y?=w210:bool)
        n182 = case shown="True" w209 {
          frame #0 {
          }
          frame #1 {
            n183 = stacked-sequence {
              frame #0 {
                n184 = local read "# Spannungsschritte"() -> (w218:i32[])
                n185 = Index Array(array=w218, index #1=0 ("Index"), index #2=1 ("Index")) -> (element #1=w215:i32, element #2=w214:i32)
                n186 = for "Schleife für Tip-Spannung" {
                  N: w215 -> [_]
                  tunnel: w214 -> [w219]
                  i -> [w220]
                  n187 = local read "Spannungsscan läuft"() -> (w221:bool)
                  n188 = case shown="True" w221 {
                    tunnel: w220 -> [_ w223]
                    tunnel: w219 -> [_ w222]
                    frame #0 {
                    }
                    frame #1 {
                      n189 = stacked-sequence {
                        tunnel: w223 -> [w225 _]
                        tunnel: w222 -> [w224 _]
                        frame #0 {
                          n190 = for "Schleife für Suppressor-Spannung" {
                            N: w224 -> [_]
                            tunnel: w225 -> [w227]
                            i -> [w226]
                            n191 = local read "Spannungsscan läuft"() -> (w228:bool)
                            n192 = case shown="True" w228 {
                              tunnel: w227 -> [_ w230]
                              tunnel: w226 -> [_ w229]
                              frame #0 {
                              }
                              frame #1 {
                                n193 = stacked-sequence {
                                tunnel: w230 -> [_ _ w272 _]
                                tunnel: w229 -> [_ _ w271 _]
                                frame #0 {
                                n194 = local read "ROI"() -> (w236:i32[])
                                n195 = local write "Summierte Helligkeit (a.u.)"(u64 0 ("Summierte Helligkeit (a.u.)")) -> ()
                                n196 = local read "Aktueller Messschritt"() -> (w233:i32)
                                n197 = Index Array(array=w236, index #1=0 ("Index"), index #2=1 ("Index")) -> (element #1=w240:i32, element #2=w239:i32)
                                n198 = Initialize Array(u64 0 ("Element"), w239, w240) -> (w234:u64[][])
                                n199 = Increment(x=w233) -> (x+1=w232:i32)
                                n200 = local write "Gemitteltes Bild"(w234) -> ()
                                n201 = local write "Aktueller Messschritt"(w232) -> ()
                                }
                                frame #1 {
                                n202 = local read "# Bilder/Messschritt"() -> (w244:i32)
                                n203 = local read "Detektionskamera"() -> (w247:T4)
                                n204 = local read "Einzelbilder speichern"() -> (w242:bool)
                                n205 = call "camera_acquisition_sequence.vi"("Session In"=w247, "Desired image number"=w244) -> ("Image Array"=w241:T3[], "error out"=w246:errorcluster)  [unwired: 2 in, 1 out]
                                n206 = case shown="True" w242 {
                                tunnel: w246 -> [w249 w257]
                                tunnel: [w249 w256] -> w245
                                tunnel: w244 -> [w248 w255]
                                tunnel: [w248 w255] -> w243
                                tunnel: w241 -> [_ w254]
                                frame #0 {
                                }
                                frame #1 {
                                n207 = local read "Aktueller Messschritt"() -> (w260:i32)
                                n208 = local read "Save folder"() -> (w252:string)
                                n209 = Concatenate Strings(w252, "Einzelbilder\\" ("String")) -> (w250:string)
                                n210 = Format Into String(format string="%05.0f" ("Format-String"), initial string="#" ("Eingangs-String"), w260) -> (resulting string=w253:string)  [unwired: 1 in, 1 out]
                                n211 = call "save images.vi"("Save Folder"=w250, "File name prefix"=w253, "Array"=w254, "error out 2"=w257, "Bilder/Messschritt"=w255) -> ("error out"=w256:errorcluster)
                                }
                                }
                                n212 = for {
                                N: w243 -> [_]
                                tunnel: w245 -> [w266]
                                tunnel: w241 -> [w264] mode=indexing
                                n213 = call "IMAQ ImageToArray"("error in (no error)"=w266, "Image"=w264) -> ("error out"=w265:errorcluster, "Image Pixels (U8)"=w263:u8[][])  [unwired: 2 in, 3 out]
                                n214 = local read "Gemitteltes Bild"() -> (w261:u64[][])
                                n215 = To Unsigned Quad Integer(1:w263) -> (0:w268:u64[][])
                                n216 = local read "Summierte Helligkeit (a.u.)"() -> (w269:u64)
                                n217 = local write "Fehler (Ausgang)"(w265) -> ()
                                n218 = Add Array Elements(numeric array=w268) -> (sum=w267:u64)
                                n219 = Add(x=w261, y=w263) -> (x+y=w262:u64[][])
                                n220 = local write "Gemitteltes Bild"(w262) -> ()
                                n221 = Add(x=w267, y=w269) -> (x+y=w270:u64)
                                n222 = local write "Summierte Helligkeit (a.u.)"(w270) -> ()
                                }
                                }
                                frame #2 {
                                n223 = local read "# Bilder/Messschritt"() -> (w278:i32)
                                n224 = local read "Gemitteltes Bild"() -> (w276:u64[][])
                                n225 = local read "Gemittelte Bilder speichern"() -> (w282:bool)
                                n226 = local read "2D-Intensitätsverteilung (MCP)"() -> (w275:dbl[][])
                                n227 = local read "Image Display"() -> (w280:T3)
                                n228 = local read "Summierte Helligkeit (a.u.)"() -> (w273:u64)
                                n229 = Divide(x=w276, y=w278) -> (x/y=w277:dbl[][])
                                n230 = call "IMAQ ArrayToImage"("Image Pixels (U8)"=w277, "Image"=w280) -> ("Image Out"=w279:T3)  [unwired: 8 in, 1 out]
                                n231 = case shown="True" w282 {
                                tunnel: w279 -> [w283 w294]
                                tunnel: [w283 w285] -> w281
                                frame #0 {
                                }
                                frame #1 {
                                n232 = local read "Aktueller Messschritt"() -> (w289:i32)
                                n233 = local read "Save folder"() -> (w291:string)
                                n234 = Format Into String(format string="%05.0f" ("Format-String"), initial string="#" ("Eingangs-String"), w289) -> (resulting string=w288:string)  [unwired: 1 in, 1 out]
                                n235 = Concatenate Strings(w291, "Gemittelte Bilder\\" ("String"), w288, ".png" ("String")) -> (w287:string)
                                n236 = String To Path(string=w287) -> (path=w286:path)
                                n237 = call-poly "IMAQ Write File 2"("File Path"=w286, "Image"=w294) -> ("Image Out (duplicate)"=w285:T3)  [unwired: 8 in, 1 out]
                                }
                                }
                                n238 = Replace Array Subset(array=w275, new element=w273, index (row)=w272, index (col)=w271) -> (w274:dbl[][])
                                n239 = local write "2D-Intensitätsverteilung (MCP)"(w274) -> ()
                                n240 = local write "Image Display"(w281) -> ()
                                }
                                frame #3 {
                                n241 = flat-sequence {
                                frame #0 {
                                n242 = local read "Aktuelle Spannung [V]"() -> (w297:dbl[])
                                n243 = local read "Spannungsschritt [V]"() -> (w301:dbl[])
                                n244 = Index Array(array=w297, index=1 ("Index")) -> (element=w299:dbl)
                                n245 = Index Array(array=w301, index=1 ("Index")) -> (element=w300:dbl)
                                n246 = Add(x=w299, y=w300) -> (x+y=w295:dbl)
                                n247 = call "HV_power_supply_set_voltage.vi"("Desired output voltage in V (HV power supply)"=w295, "Channel of HV power supply"=refnum<k21> "Dev0/Ao0") -> ("error out"=w304:errorcluster)  [unwired: 8 in]
                                n248 = Replace Array Subset(array=w297, new element=w295, index=1 ("Index")) -> (w296:dbl[])
                                n249 = local write "Fehler (Ausgang)"(w304) -> ()
                                n250 = local write "Suppressor-Spannung [V]"(w295) -> ()
                                n251 = local write "Aktuelle Spannung [V]"(w296) -> ()
                                }
                                frame #1 {
                                # "Wartezeit für\nneue Spannung"
                                n252 = Wait (ms)(milliseconds to wait=u32 200 ("Zu wartende ms")) -> ()  [unwired: 1 out]
                                }
                                frame #2 {
                                n253 = local read "Aktueller Messschritt"() -> (w308:i32)
                                n254 = local read "Start time [ms]"() -> (w310:timestamp)
                                n255 = local read "# Messschritte"() -> (w309:i32)
                                n256 = call "estimate_stopp_time.vi"("Aktueller Messschritt"=w308, "# Messschritte"=w309, "Startzeit"=w310) -> ("Stopp Zeit"=w307:string)  [unwired: 8 in]
                                n257 = local write "Geschätzte Messzeit"(w307) -> ()
                                }
                                }
                                }
                                }
                              }
                            }
                          }
                        }
                        frame #1 {
                          n258 = flat-sequence {
                            frame #0 {
                              n259 = local read "Spannungsstart [V]"() -> (w316:dbl[])
                              n260 = local read "Aktuelle Spannung [V]"() -> (w318:dbl[])
                              n261 = Index Array(array=w316, index=1 ("Index")) -> (element=w311:dbl)
                              n262 = call "HV_power_supply_set_voltage.vi"("Desired output voltage in V (HV power supply)"=w311, "Channel of HV power supply"=refnum<k21> "Dev0/Ao0") -> ("error out"=w312:errorcluster)  [unwired: 8 in]
                              n263 = local write "Suppressor-Spannung [V]"(w311) -> ()
                              n264 = Replace Array Subset(array=w318, new element=w311, index=1 ("Index")) -> (w314:dbl[])
                              n265 = local write "Fehler (Ausgang)"(w312) -> ()
                              n266 = local write "Aktuelle Spannung [V]"(w314) -> ()
                            }
                            frame #1 {
                              n267 = local read "Aktuelle Spannung [V]"() -> (w321:dbl[])
                              n268 = local read "Spannungsschritt [V]"() -> (w325:dbl[])
                              n269 = Index Array(array=w321, index=0 ("Index")) -> (element=w323:dbl)
                              n270 = Index Array(array=w325, index=0 ("Index")) -> (element=w324:dbl)
                              n271 = Add(x=w323, y=w324) -> (x+y=w319:dbl)
                              n272 = call "HV_power_supply_set_voltage.vi"("Desired output voltage in V (HV power supply)"=w319, "Channel of HV power supply"=refnum<k21> "Dev0/Ao1") -> ("error out"=w328:errorcluster)  [unwired: 8 in]
                              n273 = local write "Tip-Spannung [V]"(w319) -> ()
                              n274 = local write "Fehler (Ausgang)"(w328) -> ()
                              n275 = Replace Array Subset(array=w321, new element=w319, index=0 ("Index")) -> (w320:dbl[])
                              n276 = local write "Aktuelle Spannung [V]"(w320) -> ()
                            }
                            frame #2 {
                              # "Wartezeit für\nStartspannung"
                              n277 = Wait (ms)(milliseconds to wait=u32 6000 ("Zu wartende ms")) -> ()  [unwired: 1 out]
                            }
                          }
                        }
                      }
                    }
                  }
                }
              }
              frame #1 {
                n278 = local read "Spannungsscan läuft"() -> (w331:bool)
                n279 = case shown="True" w331 {
                  frame #0 {
                    n280 = flat-sequence {
                      frame #0 {
                        # "Zur Ausgangsposition zurückfahren"
                        n281 = local read "Spannungsstart [V]"() -> (w332:dbl[])
                        n282 = local read "Spannungsstart [V]"() -> (w337:dbl[])
                        n283 = local read "Detektionskamera"() -> (w344:T4)
                        n284 = local read "Buffer Interval"() -> (w343:u32)
                        n285 = local write "Aktuelle Spannung [V]"(w332) -> ()
                        n286 = call "camera_create_configuration.vi"("BufferInterval"=w343, "Session Out 2"=w344) -> ("Fehler (Ausgang)"=w338:errorcluster, "Ereignisregistrierung (Referenz)"=w345:refnum<event-registration>)  [unwired: 1 in, 1 out]
                        n287 = Index Array(array=w337, index #1=0 ("Index"), index #2=1 ("Index")) -> (element #1=w333:dbl, element #2=w334:dbl)
                        n288 = local write "Tip-Spannung [V]"(w333) -> ()
                        n289 = local write "Suppressor-Spannung [V]"(w334) -> ()
                        n290 = local write "Ereignis: FrameDone?"(w345) -> ()
                        n291 = call "HV_power_supply_set_voltage.vi"("error in"=w338, "Desired output voltage in V (HV power supply)"=w334, "Channel of HV power supply"=refnum<k21> "Dev0/Ao0") -> ("error out"=w340:errorcluster)  [unwired: 7 in]
                        n292 = call "HV_power_supply_set_voltage.vi"("error in"=w340, "Desired output voltage in V (HV power supply)"=w333, "Channel of HV power supply"=refnum<k21> "Dev0/Ao1") -> ("error out"=w339:errorcluster)  [unwired: 7 in]
                        n293 = local write "Fehler (Ausgang)"(w339) -> ()
                      }
                    }
                  }
                  frame #1 {
                    w347 = FALSE ("Spannungsscan läuft")
                    n294 = local read "Summierte Helligkeit speichern"() -> (w351:bool)
                    n295 = local write "Spannungsscan läuft"(w347) -> ()
                    n296 = local write "Spannungsscan ON/OFF"(w347) -> ()
                    n297 = flat-sequence {
                      frame #0 {
                        # "Zur Ausgangsposition zurückfahren"
                        n298 = local read "Spannungsstart [V]"() -> (w352:dbl[])
                        n299 = local read "Spannungsstart [V]"() -> (w357:dbl[])
                        n300 = local read "Detektionskamera"() -> (w364:T4)
                        n301 = local read "Buffer Interval"() -> (w363:u32)
                        n302 = local write "Aktuelle Spannung [V]"(w352) -> ()
                        n303 = call "camera_create_configuration.vi"("BufferInterval"=w363, "Session Out 2"=w364) -> ("Fehler (Ausgang)"=w358:errorcluster, "Ereignisregistrierung (Referenz)"=w365:refnum<event-registration>)  [unwired: 1 in, 1 out]
                        n304 = Index Array(array=w357, index #1=0 ("Index"), index #2=1 ("Index")) -> (element #1=w353:dbl, element #2=w354:dbl)
                        n305 = local write "Tip-Spannung [V]"(w353) -> ()
                        n306 = local write "Suppressor-Spannung [V]"(w354) -> ()
                        n307 = local write "Ereignis: FrameDone?"(w365) -> ()
                        n308 = call "HV_power_supply_set_voltage.vi"("error in"=w358, "Desired output voltage in V (HV power supply)"=w354, "Channel of HV power supply"=refnum<k21> "Dev0/Ao0") -> ("error out"=w360:errorcluster)  [unwired: 7 in]
                        n309 = call "HV_power_supply_set_voltage.vi"("error in"=w360, "Desired output voltage in V (HV power supply)"=w353, "Channel of HV power supply"=refnum<k21> "Dev0/Ao1") -> ("error out"=w359:errorcluster)  [unwired: 7 in]
                        n310 = local write "Fehler (Ausgang)"(w359) -> ()
                      }
                    }
                    n311 = case shown="True" w351 {
                      frame #0 {
                      }
                      frame #1 {
                        w366 = 1 ("Index")
                        w378 = 0 ("Index")
                        n312 = local read "Spannungsschritt [V]"() -> (w376:dbl[])
                        n313 = local read "# Spannungsschritte"() -> (w377:i32[])
                        n314 = local read "Spannungsstart [V]"() -> (w375:dbl[])
                        n315 = local read "Save folder"() -> (w367:string)
                        n316 = local read "2D-Intensitätsverteilung (MCP)"() -> (w384:dbl[][])
                        n317 = Index Array(array=w377, index #1=w378, index #2=w366) -> (element #1=w372:i32, element #2=w368:i32)
                        n318 = Index Array(array=w375, index #1=w378, index #2=w366) -> (element #1=w374:dbl, element #2=w370:dbl)
                        n319 = Index Array(array=w376, index #1=w378, index #2=w366) -> (element #1=w373:dbl, element #2=w369:dbl)
                        n320 = call "create_axis_vector_file.vi"("Save folder"=w367, "Dateiname"="yAchse.dat", "Start"=w370, "Schrittlänge"=w369, "# Schritte"=w368) -> ()  [unwired: 11 in]
                        n321 = call "create_axis_vector_file.vi"("Save folder"=w367, "Dateiname"="xAchse.dat" ("Save folder"), "Start"=w374, "Schrittlänge"=w373, "# Schritte"=w372) -> ()  [unwired: 11 in]
                        n322 = Concatenate Strings(w367, "\\" ("String"), "2D_Intensitaetsverteilung_MCP.dat" ("String")) -> (w381:string)
                        n323 = String To Path(string=w381) -> (path=w382:path)
                        n324 = call-poly <vilib>:"Write To Spreadsheet File.vi"("format (%.3f)"="%.;%8.0f", "2D data"=w384, "file path (dialog if empty)"=w382) -> ()  [unwired: 5 in, 1 out]
                      }
                    }
                    n325 = local read "2D-Intensitätsverteilung (MCP)"() -> (w350:dbl[][])
                    n326 = control-ref of="2D-Intensitätsverteilung (MCP)"() -> (w346:refnum<vi>)
                    n327 = Array Max & Min(array=w350) -> (max value=w349:dbl, min value=w348:dbl)  [unwired: 2 out]
                    n328 = property class="IntGraph (strikt)"(reference=w346, "ZScale.Maximum"=w349, "ZScale.Minimum"=w348) -> ()  [unwired: 1 in, 2 out]
                  }
                }
              }
            }
          }
        }
      }
      n329 = while "x-U-Scan Schleife" {
        stop <- w60 stop-if-true
        n330 = local read "Fehler (Ausgang)"() -> (w61:errorcluster)
        n331 = local read "x-U-Scan läuft"() -> (w59:bool)
        n332 = local read "Programm beenden"() -> (w63:bool)
        n333 = Unbundle By Name(w61) -> ("status"=w62:bool)
        n334 = case shown="True" w59 {
          frame #0 {
          }
          frame #1 {
            n335 = stacked-sequence {
              frame #0 {
                n336 = local read "# x-U-Scan Rasterschritte"() -> (w64:i32)
                n337 = for "Schleife für Raumkoordinate" {
                  N: w64 -> [_]
                  i -> [w65]
                  n338 = local read "x-U-Scan läuft"() -> (w66:bool)
                  n339 = case shown="True" w66 {
                    tunnel: w65 -> [_ w67]
                    frame #0 {
                    }
                    frame #1 {
                      n340 = stacked-sequence {
                        tunnel: w67 -> [w69 _]
                        frame #0 {
                          n341 = local read "# x-U-Scan Spannungsschritte"() -> (w68:i32)
                          n342 = for "Schleife für Spannungskoordinate" {
                            N: w68 -> [_]
                            tunnel: w69 -> [w71]
                            i -> [w70]
                            n343 = local read "x-U-Scan läuft"() -> (w72:bool)
                            n344 = case shown="True" w72 {
                              tunnel: w71 -> [_ w74]
                              tunnel: w70 -> [_ w73]
                              frame #0 {
                              }
                              frame #1 {
                                n345 = stacked-sequence {
                                tunnel: w74 -> [_ _ w116 _]
                                tunnel: w73 -> [_ _ w115 _]
                                frame #0 {
                                n346 = local read "ROI"() -> (w80:i32[])
                                n347 = local write "Summierte Helligkeit (a.u.)"(u64 0 ("Summierte Helligkeit (a.u.)")) -> ()
                                n348 = local read "Aktueller Messschritt"() -> (w77:i32)
                                n349 = Index Array(array=w80, index #1=0 ("Index"), index #2=1 ("Index")) -> (element #1=w84:i32, element #2=w83:i32)
                                n350 = Initialize Array(u64 0 ("Element"), w83, w84) -> (w78:u64[][])
                                n351 = Increment(x=w77) -> (x+1=w76:i32)
                                n352 = local write "Gemitteltes Bild"(w78) -> ()
                                n353 = local write "Aktueller Messschritt"(w76) -> ()
                                }
                                frame #1 {
                                n354 = local read "# Bilder/Messschritt"() -> (w88:i32)
                                n355 = local read "Detektionskamera"() -> (w91:T4)
                                n356 = local read "Einzelbilder speichern"() -> (w86:bool)
                                n357 = call "camera_acquisition_sequence.vi"("Session In"=w91, "Desired image number"=w88) -> ("Image Array"=w85:T3[], "error out"=w90:errorcluster)  [unwired: 2 in, 1 out]
                                n358 = case shown="True" w86 {
                                tunnel: w90 -> [w93 w101]
                                tunnel: [w93 w100] -> w89
                                tunnel: w88 -> [w92 w99]
                                tunnel: [w92 w99] -> w87
                                tunnel: w85 -> [_ w98]
                                frame #0 {
                                }
                                frame #1 {
                                n359 = local read "Aktueller Messschritt"() -> (w104:i32)
                                n360 = local read "Save folder"() -> (w96:string)
                                n361 = Concatenate Strings(w96, "Einzelbilder\\" ("String")) -> (w94:string)
                                n362 = Format Into String(format string="%05.0f" ("Format-String"), initial string="#" ("Eingangs-String"), w104) -> (resulting string=w97:string)  [unwired: 1 in, 1 out]
                                n363 = call "save images.vi"("Save Folder"=w94, "File name prefix"=w97, "Array"=w98, "error out 2"=w101, "Bilder/Messschritt"=w99) -> ("error out"=w100:errorcluster)
                                }
                                }
                                n364 = for {
                                N: w87 -> [_]
                                tunnel: w89 -> [w110]
                                tunnel: w85 -> [w108] mode=indexing
                                n365 = call "IMAQ ImageToArray"("error in (no error)"=w110, "Image"=w108) -> ("error out"=w109:errorcluster, "Image Pixels (U8)"=w107:u8[][])  [unwired: 2 in, 3 out]
                                n366 = local read "Gemitteltes Bild"() -> (w105:u64[][])
                                n367 = To Unsigned Quad Integer(1:w107) -> (0:w112:u64[][])
                                n368 = local read "Summierte Helligkeit (a.u.)"() -> (w113:u64)
                                n369 = local write "Fehler (Ausgang)"(w109) -> ()
                                n370 = Add Array Elements(numeric array=w112) -> (sum=w111:u64)
                                n371 = Add(x=w105, y=w107) -> (x+y=w106:u64[][])
                                n372 = local write "Gemitteltes Bild"(w106) -> ()
                                n373 = Add(x=w111, y=w113) -> (x+y=w114:u64)
                                n374 = local write "Summierte Helligkeit (a.u.)"(w114) -> ()
                                }
                                }
                                frame #2 {
                                n375 = local read "# Bilder/Messschritt"() -> (w122:i32)
                                n376 = local read "Gemitteltes Bild"() -> (w120:u64[][])
                                n377 = local read "2D-Intensitätsverteilung (MCP)"() -> (w119:dbl[][])
                                n378 = local read "Summierte Helligkeit (a.u.)"() -> (w117:u64)
                                n379 = local read "Gemittelte Bilder speichern"() -> (w126:bool)
                                n380 = local read "Image Display"() -> (w124:T3)
                                n381 = Divide(x=w120, y=w122) -> (x/y=w121:dbl[][])
                                n382 = call "IMAQ ArrayToImage"("Image Pixels (U8)"=w121, "Image"=w124) -> ("Image Out"=w123:T3)  [unwired: 8 in, 1 out]
                                n383 = Replace Array Subset(array=w119, new element=w117, index (row)=w116, index (col)=w115) -> (w118:dbl[][])
                                n384 = case shown="True" w126 {
                                tunnel: w123 -> [w127 w138]
                                tunnel: [w127 w129] -> w125
                                frame #0 {
                                }
                                frame #1 {
                                n385 = local read "Aktueller Messschritt"() -> (w133:i32)
                                n386 = local read "Save folder"() -> (w135:string)
                                n387 = Format Into String(format string="%05.0f" ("Format-String"), initial string="#" ("Eingangs-String"), w133) -> (resulting string=w132:string)  [unwired: 1 in, 1 out]
                                n388 = Concatenate Strings(w135, "Gemittelte Bilder\\" ("String"), w132, ".png" ("String")) -> (w131:string)
                                n389 = String To Path(string=w131) -> (path=w130:path)
                                n390 = call-poly "IMAQ Write File 2"("File Path"=w130, "Image"=w138) -> ("Image Out (duplicate)"=w129:T3)  [unwired: 8 in, 1 out]
                                }
                                }
                                n391 = local write "2D-Intensitätsverteilung (MCP)"(w118) -> ()
                                n392 = local write "Image Display"(w125) -> ()
                                }
                                frame #3 {
                                n393 = flat-sequence {
                                frame #0 {
                                n394 = local read "x-U-Scan aktuelle Spannung [V]"() -> (w141:dbl)
                                n395 = local read "x-U-Scan Spannungsschritt [V]"() -> (w142:dbl)
                                n396 = local read "Spannungskanal"() -> (w140:refnum<k21>)
                                n397 = Add(x=w141, y=w142) -> (x+y=w139:dbl)
                                n398 = local write "x-U-Scan aktuelle Spannung [V]"(w139) -> ()
                                n399 = call "HV_power_supply_set_voltage.vi"("Desired output voltage in V (HV power supply)"=w139, "Channel of HV power supply"=w140) -> ("error out"=w143:errorcluster)  [unwired: 8 in]
                                n400 = local write "Fehler (Ausgang)"(w143) -> ()
                                }
                                frame #1 {
                                # "Wartezeit für\nneue Spannung"
                                n401 = Wait (ms)(milliseconds to wait=u32 200 ("Zu wartende ms")) -> ()  [unwired: 1 out]
                                }
                                frame #2 {
                                n402 = local read "Aktueller Messschritt"() -> (w146:i32)
                                n403 = local read "Start time [ms]"() -> (w148:timestamp)
                                n404 = local read "# Messschritte"() -> (w147:i32)
                                n405 = call "estimate_stopp_time.vi"("Aktueller Messschritt"=w146, "# Messschritte"=w147, "Startzeit"=w148) -> ("Stopp Zeit"=w145:string)  [unwired: 8 in]
                                n406 = local write "Geschätzte Messzeit"(w145) -> ()
                                }
                                }
                                }
                                }
                              }
                            }
                          }
                        }
                        frame #1 {
                          n407 = flat-sequence {
                            frame #0 {
                              n408 = local read "x-U-Scan Spannungsstart [V]"() -> (w149:dbl)
                              n409 = local read "Spannungskanal"() -> (w150:refnum<k21>)
                              n410 = local write "x-U-Scan aktuelle Spannung [V]"(w149) -> ()
                              n411 = call "HV_power_supply_set_voltage.vi"("Desired output voltage in V (HV power supply)"=w149, "Channel of HV power supply"=w150) -> ("error out"=w151:errorcluster)  [unwired: 8 in]
                              n412 = local write "Fehler (Ausgang)"(w151) -> ()
                            }
                            frame #1 {
                              # "Fahre nächste Position an"
                              n413 = local read "x-U-Scan Rasterschritt [µm]"() -> (w156:dbl)
                              n414 = local read "Achs-ID"() -> (w155:i32)
                              n415 = Decrement(x=w155) -> (x-1=w154:i32)
                              n416 = call "stage_move_axis_relative.vi"("Achse"=w155, "Schrittweite [µm]"=w156) -> ("xyz-Position OUT [mm]"=w153:dbl[])  [unwired: 1 in, 2 out]
                              n417 = Index Array(array=w153, index=w154) -> (element=w152:dbl)
                              n418 = local write "x-U-Scan aktuelle Position [mm]"(w152) -> ()
                            }
                            frame #2 {
                              # "Wartezeit für\nStartspannung"
                              n419 = Wait (ms)(milliseconds to wait=u32 6000 ("Zu wartende ms")) -> ()  [unwired: 1 out]
                            }
                          }
                        }
                      }
                    }
                  }
                }
              }
              frame #1 {
                n420 = local read "x-U-Scan läuft"() -> (w158:bool)
                n421 = case shown="True" w158 {
                  frame #0 {
                    n422 = flat-sequence {
                      frame #0 {
                        # "Zur Ausgangsposition zurückfahren"
                        n423 = local read "x-U-Scan Startposition [mm]"() -> (w159:dbl)
                        n424 = local read "Aktuelle xyz-Position [mm]"() -> (w162:dbl[])
                        n425 = local read "x-U-Scan Spannungsstart [V]"() -> (w166:dbl)
                        n426 = local read "Buffer Interval"() -> (w169:u32)
                        n427 = local read "Achs-ID"() -> (w160:i32)
                        n428 = Decrement(x=w160) -> (x-1=w161:i32)
                        n429 = local read "Detektionskamera"() -> (w170:T4)
                        n430 = Replace Array Subset(array=w162, new element=w159, index=w161) -> (w163:dbl[])
                        n431 = local read "Spannungskanal"() -> (w167:refnum<k21>)
                        n432 = local write "x-U-Scan aktuelle Spannung [V]"(w166) -> ()
                        n433 = call "stage_move_axis_absolute.vi"("Ziel xyz IN [mm]"=w163, "Achse"=w160) -> ("error out"=w164:errorcluster)  [unwired: 1 in, 2 out]
                        n434 = call "camera_create_configuration.vi"("error in"=w164, "BufferInterval"=w169, "Session Out 2"=w170) -> ("Fehler (Ausgang)"=w168:errorcluster, "Ereignisregistrierung (Referenz)"=w171:refnum<event-registration>)  [unwired: 1 out]
                        n435 = local write "Ereignis: FrameDone?"(w171) -> ()
                        n436 = call "HV_power_supply_set_voltage.vi"("error in"=w168, "Desired output voltage in V (HV power supply)"=w166, "Channel of HV power supply"=w167) -> ("error out"=w165:errorcluster)  [unwired: 7 in]
                        n437 = local write "Fehler (Ausgang)"(w165) -> ()
                      }
                    }
                  }
                  frame #1 {
                    w173 = FALSE ("Spannungsscan läuft")
                    n438 = local read "Summierte Helligkeit speichern"() -> (w177:bool)
                    n439 = flat-sequence {
                      frame #0 {
                        # "Zur Ausgangsposition zurückfahren"
                        n440 = local read "Start xyz-Position [mm]"() -> (w182:dbl[])
                        n441 = local read "x-U-Scan Spannungsstart [V]"() -> (w187:dbl)
                        n442 = local read "x-U-Scan Spannungsstart [V]"() -> (w185:dbl)
                        n443 = local read "Detektionskamera"() -> (w190:T4)
                        n444 = local read "Achs-ID"() -> (w179:i32)
                        n445 = local read "Buffer Interval"() -> (w189:u32)
                        n446 = local read "Spannungskanal"() -> (w186:refnum<k21>)
                        n447 = Decrement(x=w179) -> (x-1=w180:i32)
                        n448 = call "stage_move_axis_absolute.vi"("Ziel xyz IN [mm]"=w182, "Achse"=w179) -> ("error out"=w183:errorcluster, "Ziel xyz OUT [mm]"=w181:dbl[])  [unwired: 1 in, 1 out]
                        n449 = call "camera_create_configuration.vi"("error in"=w183, "BufferInterval"=w189, "Session Out 2"=w190) -> ("Fehler (Ausgang)"=w184:errorcluster, "Ereignisregistrierung (Referenz)"=w191:refnum<event-registration>)  [unwired: 1 out]
                        n450 = Index Array(array=w181, index=w180) -> (element=w178:dbl)
                        n451 = local write "x-U-Scan aktuelle Spannung [V]"(w185) -> ()
                        n452 = local write "x-U-Scan aktuelle Position [mm]"(w178) -> ()
                        n453 = local write "Ereignis: FrameDone?"(w191) -> ()
                        n454 = call "HV_power_supply_set_voltage.vi"("error in"=w184, "Desired output voltage in V (HV power supply)"=w185, "Channel of HV power supply"=w186) -> ("error out"=w188:errorcluster)  [unwired: 7 in]
                        n455 = local write "x-U-Scan aktuelle Spannung [V]"(w187) -> ()
                        n456 = local write "Fehler (Ausgang)"(w188) -> ()
                      }
                    }
                    n457 = local read "2D-Intensitätsverteilung (MCP)"() -> (w176:dbl[][])
                    n458 = local write "x-U-Scan läuft"(w173) -> ()
                    n459 = local write "x-U-Scan ON/OFF"(w173) -> ()
                    n460 = case shown="True" w177 {
                      frame #0 {
                      }
                      frame #1 {
                        n461 = local read "x-U-Scan Rasterschritt [µm]"() -> (w194:dbl)
                        n462 = local read "x-U-Scan Spannungsschritt [V]"() -> (w198:dbl)
                        n463 = local read "# x-U-Scan Spannungsschritte"() -> (w197:i32)
                        n464 = local read "x-U-Scan Spannungsstart [V]"() -> (w199:dbl)
                        n465 = local read "x-U-Scan Startposition [mm]"() -> (w195:dbl)
                        n466 = local read "# x-U-Scan Rasterschritte"() -> (w196:i32)
                        n467 = local read "Save folder"() -> (w201:string)
                        n468 = local read "2D-Intensitätsverteilung (MCP)"() -> (w207:dbl[][])
                        n469 = Divide(x=w194, y=1000.0) -> (x/y=w193:dbl)
                        n470 = call "create_axis_vector_file.vi"("Save folder"=w201, "Dateiname"="yAchse.dat", "Start"=w199, "Schrittlänge"=w198, "# Schritte"=w197) -> ()  [unwired: 11 in]
                        n471 = call "create_axis_vector_file.vi"("Save folder"=w201, "Dateiname"="xAchse.dat", "Start"=w195, "Schrittlänge"=w193, "# Schritte"=w196) -> ()  [unwired: 11 in]
                        n472 = Concatenate Strings(w201, "\\" ("String"), "2D_Intensitaetsverteilung_MCP.dat" ("String")) -> (w204:string)
                        n473 = String To Path(string=w204) -> (path=w205:path)
                        n474 = call-poly <vilib>:"Write To Spreadsheet File.vi"("format (%.3f)"="%.;%8.0f", "2D data"=w207, "file path (dialog if empty)"=w205) -> ()  [unwired: 5 in, 1 out]
                      }
                    }
                    n475 = control-ref of="2D-Intensitätsverteilung (MCP)"() -> (w172:refnum<vi>)
                    n476 = Array Max & Min(array=w176) -> (max value=w175:dbl, min value=w174:dbl)  [unwired: 2 out]
                    n477 = property class="IntGraph (strikt)"(reference=w172, "ZScale.Maximum"=w175, "ZScale.Minimum"=w174) -> ()  [unwired: 1 in, 2 out]
                  }
                }
              }
            }
          }
        }
        n478 = Or(x=w62, y=w63) -> (x .or. y?=w60:bool)
      }
      n479 = while "Mess-Schleife" {
        tunnel: w58 -> [w439]
        i -> [w437]
        stop <- w438 stop-if-true
        n480 = event "Scan-Ereignisse" shown="[1] \"Rasterung ON/OFF\": Wertänderung" {
          selector: w439 -> [_ _ _ _ _ _ _]
          dyn-events: _ -> [_ _ _ _ _ _ _]
          timeout: 1000 -> [_ _ _ _ _ _ _]
          event #0 {
            n481 = event-data() -> ()  [unwired: 1 in, 2 out]
          }
          event #1 {
            n482 = event-data() -> ("NewVal"=w446:bool)  [unwired: 1 in]
            n483 = local read "Kamera"() -> (w445:bool)
            n484 = And(x=w445, y=w446) -> (x .and. y?=w444:bool)
            n485 = case shown="True" w444 {
              frame #0 {
                n486 = local write "Rasterung läuft"(FALSE ("Rasterung läuft")) -> ()
              }
              frame #1 {
                n487 = stacked-sequence {
                  frame #0 {
                    n488 = flat-sequence {
                      tunnel: [w458] -> w448
                      tunnel: w448 -> [w513]
                      frame #0 {
                        n489 = local read "# Bilder/Messschritt"() -> (w464:i32)
                        n490 = local read "Rasterweite [µm]"() -> (w469:dbl[])
                        n491 = local read "# Rasterschritte"() -> (w471:i32[])
                        n492 = control-ref of="Rasterart"() -> (w467:refnum<vi>)
                        n493 = local read "ROI"() -> (w452:i32[])
                        n494 = property class="Enum (strikt)"(reference=w467) -> ("RingText.Text"=w453:string)  [unwired: 1 in, 2 out]
                        n495 = local read "Rasterart"() -> (w472:T2)
                        n496 = control-ref of="Shutter time (ms)"() -> (w466:refnum<vi>)
                        n497 = call "stage_get_current_xyz.vi"() -> ("Aktuelle xyz-Position OUT [mm]"=w457:dbl[])  [unwired: 3 in, 1 out]
                        n498 = case shown="\"Linescan(x)\", Voreinstellung" w472 {
                          tunnel: w471 -> [w480 w496 w501 w510]
                          tunnel: [w479 w495 w502 w509] -> w470
                          tunnel: w469 -> [w478 w486 w498 w506]
                          tunnel: [w477 w485 w497 w505] -> w468
                          frame #0 {
                            n499 = Replace Array Subset(array=w478, new element #1=0.0 ("Neues Element/Teil-Array"), index #1=1 ("Index"), new element #2=0.0 ("Neues Element/Teil-Array"), index #2=2 ("Index")) -> (w477:dbl[])
                            n500 = Replace Array Subset(array=w480, new element #1=1 ("Neues Element/Teil-Array"), index #1=1 ("Index"), new element #2=1 ("Neues Element/Teil-Array"), index #2=2 ("Index")) -> (w479:i32[])
                          }
                          frame #1 {
                            n501 = Replace Array Subset(array=w486, new element #1=0.0 ("Neues Element/Teil-Array"), index #1=0 ("Index"), new element #2=0.0 ("Neues Element/Teil-Array"), index #2=1 ("Index")) -> (w485:dbl[])
                            n502 = Replace Array Subset(array=w496, new element #1=1 ("Neues Element/Teil-Array"), index #1=0 ("Index"), new element #2=1 ("Neues Element/Teil-Array"), index #2=1 ("Index")) -> (w495:i32[])
                          }
                          frame #2 {
                            n503 = Replace Array Subset(array=w498, new element=0.0 ("Neues Element/Teil-Array"), index=2 ("Index")) -> (w497:dbl[])
                            n504 = Replace Array Subset(array=w501, new element=1 ("Neues Element/Teil-Array"), index=2 ("Index")) -> (w502:i32[])
                          }
                          frame #3 {
                            n505 = Replace Array Subset(array=w506, new element=0.0 ("Neues Element/Teil-Array"), index=0 ("Index")) -> (w505:dbl[])
                            n506 = Replace Array Subset(array=w510, new element=1 ("Neues Element/Teil-Array"), index=0 ("Index")) -> (w509:i32[])
                          }
                        }
                        n507 = property class="Ring (strikt)"(reference=w466) -> ("RingText.Text"=w465:string)  [unwired: 1 in, 2 out]
                        n508 = Decimal String To Number(string=w465) -> (number=w462:i32)  [unwired: 2 in, 1 out]
                        n509 = local read "P-Schirm-Spannung [V]"() -> (w456:dbl)
                        n510 = local read "Suppressor-Spannung [V]"() -> (w451:dbl)
                        n511 = local read "MCP-Spannung [V]"() -> (w455:dbl)
                        n512 = local read "Leistung (iK) [mW]"() -> (w454:dbl)
                        n513 = local read "Polarisation [°]"() -> (w459:dbl)
                        n514 = local read "Tip-Spannung [V]"() -> (w450:dbl)
                        n515 = local read "Messlogbuch"() -> (w461:path)
                        n516 = local read "Proben-ID"() -> (w460:string)
                        n517 = Get Date/Time In Seconds() -> (seconds since 1Jan1904=w449:timestamp)
                        n518 = Multiply(x=w464, y=w462) -> (x*y=w463:i32)
                        n519 = local write "Start time [ms]"(w449) -> ()
                        n520 = local write "Rasterweite [µm]"(w468) -> ()
                        n521 = local write "# Rasterschritte"(w470) -> ()
                        n522 = call "create_measure_log_entry.vi"("Messlogbuch-Pfad"=w461, "Probe"=w460, "Polarisation [°]"=w459, "Messart"=w453, "ROI"=w452, "Messungen/Messschritt"=w464, "Maximalleistung (iK) [mW]"=w454, "Tip-Spannung [V]"=w450, "Suppressor-Spannung [V]"=w451, "Zeit/Messschritt [ms]"=w462, "MCP-Spannung [V]"=w455, "Zeit/Messung [ms]"=w463, "Phosphorschirm-Spannung [V]"=w456, "xyz [mm]"=w457) -> ("Messung Nr."=w458:i32)  [unwired: 4 in, 1 out]
                      }
                      frame #1 {
                        n523 = local read "Day folder"() -> (w519:string)
                        n524 = local read "Fehler (Ausgang)"() -> (w514:errorcluster)
                        n525 = local write "Aktueller Messschritt"(0 ("Aktueller Messschritt")) -> ()
                        n526 = local read "Rasterweite [µm]"() -> (w539:dbl[])
                        n527 = local read "# Rasterschritte"() -> (w538:i32[])
                        n528 = local read "# Rasterschritte"() -> (w536:i32[])
                        n529 = local read "Einzelbilder speichern"() -> (w522:bool)
                        n530 = call "create_save_folder.vi"("Day folder"=w519, "Measuring number"=w513, "Measuring folder"="Rasterung" ("Subfolder"), "error in"=w514) -> ("Save Folder"=w518:string, "Error Out"=w517:errorcluster)  [unwired: 5 in]
                        n531 = local write "Save folder"(w518) -> ()
                        n532 = Divide(x=w539, y=w538) -> (x/y=w537:dbl[])
                        n533 = Index Array(array=w536, index #1=0 ("Index"), index #2=1 ("Index"), index #3=2 ("Index")) -> (element #1=w533:i32, element #2=w532:i32, element #3=w531:i32)
                        n534 = local read "Gemittelte Bilder speichern"() -> (w523:bool)
                        n535 = Multiply(x=w533, y=w532) -> (x*y=w530:i32)
                        n536 = local write "Rasterschritt [µm]"(w537) -> ()
                        n537 = case shown="True" w522 {
                          tunnel: w517 -> [w540 w542]
                          tunnel: [w540 w541] -> w516
                          frame #0 {
                          }
                          frame #1 {
                            n538 = local read "Save folder"() -> (w545:string)
                            n539 = Concatenate Strings(w545, "\\Einzelbilder" ("Subfolder")) -> (w543:string)
                            n540 = String To Path(string=w543) -> (path=w546:path)
                            n541 = call <vilib>:"Check if File or Folder Exists.vi"("error in (no error)"=w542, "path"=w546) -> ("error out"=w541:errorcluster, "file or folder exists?"=w547:bool, "dup path"=w548:path)  [unwired: 7 in]
                            n542 = case shown="False" w547 {
                              tunnel: w548 -> [w549 _]
                              frame #0 {
                                n543 = Create Folder(path (use dialog)=w549) -> ()  [unwired: 2 in, 3 out]
                              }
                              frame #1 {
                              }
                            }
                          }
                        }
                        n544 = local read "Kamera"() -> (w525:bool)
                        n545 = Multiply(x=w530, y=w531) -> (x*y=w529:i32)
                        n546 = local write "# Messschritte"(w529) -> ()
                        n547 = case shown="True" w523 {
                          tunnel: w516 -> [w550 w552]
                          tunnel: [w550 w551] -> w515
                          frame #0 {
                          }
                          frame #1 {
                            n548 = local read "Save folder"() -> (w556:string)
                            n549 = Concatenate Strings(w556, "\\Gemittelte Bilder" ("Subfolder")) -> (w558:string)
                            n550 = String To Path(string=w558) -> (path=w555:path)
                            n551 = call <vilib>:"Check if File or Folder Exists.vi"("error in (no error)"=w552, "path"=w555) -> ("error out"=w551:errorcluster, "file or folder exists?"=w554:bool, "dup path"=w553:path)  [unwired: 7 in]
                            n552 = case shown="False" w554 {
                              tunnel: w553 -> [w559 _]
                              frame #0 {
                                n553 = Create Folder(path (use dialog)=w559) -> ()  [unwired: 2 in, 3 out]
                              }
                              frame #1 {
                              }
                            }
                          }
                        }
                        n554 = case shown="True" w525 {
                          tunnel: [w560 w562] -> w524
                          tunnel: w515 -> [w560 w561]
                          frame #0 {
                          }
                          frame #1 {
                            n555 = local read "Ereignis: FrameDone?"() -> (w563:refnum<event-registration>)
                            n556 = local read "Detektionskamera"() -> (w564:T4)
                            n557 = call "camera_release_configuration.vi"("error in"=w561, "Session In"=w564, "Ereignisregistrierung (Referenz) 2"=w563) -> ("error out"=w562:errorcluster)  [unwired: 1 out]
                          }
                        }
                        n558 = call "stage_get_current_xyz.vi"("error in"=w524) -> ("error out"=w521:errorcluster, "Aktuelle xyz-Position OUT [mm]"=w526:dbl[])  [unwired: 2 in]
                        n559 = local write "Start xyz-Position [mm]"(w526) -> ()
                        n560 = local write "Fehler (Ausgang)"(w521) -> ()
                      }
                    }
                  }
                  frame #1 {
                    n561 = flat-sequence {
                      tunnel: [w579] -> w575
                      tunnel: [w578] -> w574
                      tunnel: [w577] -> w573
                      tunnel: [w577] -> w572
                      tunnel: [w577] -> w571
                      tunnel: [w577] -> w570
                      tunnel: [w577] -> w569
                      tunnel: [w576] -> w568
                      tunnel: [w577] -> w567
                      tunnel: [w577] -> w566
                      tunnel: [w576] -> w565
                      tunnel: w575 -> [w599]
                      tunnel: w574 -> [w598]
                      tunnel: w573 -> [w597]
                      tunnel: w572 -> [w596]
                      tunnel: w571 -> [w595]
                      tunnel: w570 -> [w594]
                      tunnel: w569 -> [w593]
                      tunnel: w568 -> [w592]
                      tunnel: w567 -> [w591]
                      tunnel: w566 -> [w590]
                      tunnel: w565 -> [w589]
                      frame #0 {
                        n562 = local read "Rasterart"() -> (w580:T2)
                        n563 = case shown="\"2D-Scan(yz)\"" w580 {
                          tunnel: [0 ("Index") 2 ("Index")] -> w576
                          tunnel: [1 ("Index") 1 ("Index")] -> w577
                          tunnel: ["x-Position [mm]" ("X-Achse.Namensbeschriftung.Text") "z-Position [mm]" ("Y-Achse.Namensbeschriftung.Text")] -> w579
                          tunnel: ["y-Position [mm]" ("Y-Achse.Namensbeschriftung.Text") "y-Position [mm]" ("X-Achse.Namensbeschriftung.Text")] -> w578
                          frame #0 {
                          }
                          frame #1 {
                          }
                        }
                      }
                      frame #1 {
                        w607 = 1000.0 ("y")
                        w626 = 1000.0 ("y")
                        n564 = local read "Rasterweite [µm]"() -> (w631:dbl[])
                        n565 = local read "# Rasterschritte"() -> (w635:i32[])
                        n566 = local read "Rasterweite [µm]"() -> (w602:dbl[])
                        n567 = local read "# Rasterschritte"() -> (w624:i32[])
                        n568 = local read "Start xyz-Position [mm]"() -> (w630:dbl[])
                        n569 = Index Array(array=w635, index #1=w592, index #2=w597) -> (element #1=w633:i32, element #2=w634:i32)
                        n570 = Index Array(array=w631, index #1=w592, index #2=w591) -> (element #1=w627:dbl, element #2=w628:dbl)
                        n571 = local read "# Rasterschritte"() -> (w609:i32[])
                        n572 = Divide(x=w627, y=w626) -> (x/y=w621:dbl)
                        n573 = Divide(x=w628, y=w626) -> (x/y=w623:dbl)
                        n574 = local read "Start xyz-Position [mm]"() -> (w603:dbl[])
                        n575 = Index Array(array=w624, index #1=w592, index #2=w596) -> (element #1=w620:i32, element #2=w622:i32)
                        n576 = Index Array(array=w602, index #1=w592, index #2=w593) -> (element #1=w606:dbl, element #2=w605:dbl)
                        n577 = Initialize Array(0.0 ("y"), w633, w634) -> (w616:dbl[][])
                        n578 = control-ref of="2D-Intensitätsverteilung (MCP)"() -> (w632:refnum<vi>)
                        n579 = Divide(x=w606, y=w607) -> (x/y=w612:dbl)
                        n580 = Divide(x=w605, y=w607) -> (x/y=w610:dbl)
                        n581 = Index Array(array=w630, index #1=w589, index #2=w590) -> (element #1=w629:dbl, element #2=w625:dbl)
                        n582 = Index Array(array=w609, index #1=w592, index #2=w595) -> (element #1=w613:i32, element #2=w611:i32)
                        n583 = local write "2D-Intensitätsverteilung (LAPD)"(w616) -> ()
                        n584 = Divide(x=w621, y=w620) -> (x/y=w619:dbl)
                        n585 = Divide(x=w623, y=w622) -> (x/y=w618:dbl)
                        n586 = local write "2D-Intensitätsverteilung (MCP)"(w616) -> ()
                        n587 = property class="IntGraph (strikt)"(reference=w632, "XScale.Offset"=w629, "XScale.Multiplier"=w619, "YScale.Offset"=w625, "YScale.Multiplier"=w618, "XScale.MinorInc"=w619, "YScale.MinorInc"=w618, "XScale.NameLbl.Text"=w599, "YScale.NameLbl.Text"=w598) -> (error out=w636:errorcluster)  [unwired: 1 in, 1 out]
                        n588 = Index Array(array=w603, index #1=w592, index #2=w594) -> (element #1=w604:dbl, element #2=w608:dbl)
                        n589 = control-ref of="2D-Intensitätsverteilung (LAPD)"() -> (w600:refnum<vi>)
                        n590 = Divide(x=w612, y=w613) -> (x/y=w614:dbl)
                        n591 = Divide(x=w610, y=w611) -> (x/y=w615:dbl)
                        n592 = property class="IntGraph (strikt)"(reference=w600, error in=w636, "XScale.Offset"=w604, "XScale.Multiplier"=w614, "YScale.Offset"=w608, "YScale.Multiplier"=w615, "XScale.MinorInc"=w614, "YScale.MinorInc"=w615, "XScale.NameLbl.Text"=w599, "YScale.NameLbl.Text"=w598) -> (error out=w601:errorcluster)  [unwired: 1 out]
                        n593 = local write "Fehler (Ausgang)"(w601) -> ()
                      }
                    }
                  }
                  frame #2 {
                    n594 = local read "Event: Rasterung gestartet?"() -> (w640:refnum<user-event>)
                    n595 = local write "Rasterung läuft"(TRUE ("x-Linsescan")) -> ()
                    n596 = local read "Aktueller Messschritt"() -> (w639:i32)
                    n597 = Generate User Event(user event=w640, event data cluster=w639) -> (user event out=w638:refnum<user-event>)  [unwired: 1 in, 1 out]
                    n598 = local write "Event: Rasterung gestartet?"(w638) -> ()
                  }
                }
              }
            }
          }
          event #2 {
            n599 = event-data() -> ()  [unwired: 1 in, 1 out]
            n600 = local read "Rasterweite [µm]"() -> (w642:dbl[])
            n601 = local read "# Rasterschritte"() -> (w653:i32[])
            n602 = Replace Array Subset(array=w642, new element #1=0 ("Neues Element/Teil-Array"), index #1=0 ("Index"), new element #2=0 ("Neues Element/Teil-Array"), index #2=1 ("Index"), new element #3=0 ("Neues Element/Teil-Array"), index #3=2 ("Index")) -> (w641:dbl[])
            n603 = Replace Array Subset(array=w653, new element #1=1 ("Neues Element/Teil-Array"), index #1=0 ("Index"), new element #2=1 ("Neues Element/Teil-Array"), index #2=1 ("Index"), new element #3=1 ("Neues Element/Teil-Array"), index #3=2 ("Index")) -> (w649:i32[])
            n604 = local write "Rasterweite [µm]"(w641) -> ()
            n605 = local write "# Rasterschritte"(w649) -> ()
          }
          event #3 {
            n606 = event-data() -> ()  [unwired: 1 in, 1 out]
            n607 = stacked-sequence {
              frame #0 {
                n608 = while "z-Schleife" {
                  i -> [w658]
                  stop <- w659 stop-if-true
                  n609 = stacked-sequence {
                    frame #0 {
                      n610 = while "x-Schleife" {
                        i -> [w667]
                        stop <- w669 stop-if-true
                        n611 = stacked-sequence {
                          frame #0 {
                            n612 = while "y-Schleife" {
                              i -> [w678]
                              stop <- w684 stop-if-true
                              # "Schleife für y-Achse"
                              n613 = stacked-sequence {
                                frame #0 {
                                # "Hier findet die Messung statt"
                                n614 = stacked-sequence {
                                frame #0 {
                                n615 = local write "LAPD Spannung (V)"(0.0 ("Transmittierte Intensität (a.u.)")) -> ()
                                n616 = local write "Summierte Helligkeit (a.u.)"(u64 0 ("Summierte Helligkeit (a.u.)")) -> ()
                                n617 = local read "ROI"() -> (w691:i32[])
                                n618 = Index Array(array=w691, index #1=0 ("Index"), index #2=1 ("Index")) -> (element #1=w687:i32, element #2=w688:i32)
                                n619 = local read "Aktueller Messschritt"() -> (w694:i32)
                                n620 = Initialize Array(u64 0 ("Element"), w688, w687) -> (w693:u64[][])
                                n621 = local write "Gemitteltes Bild"(w693) -> ()
                                n622 = Increment(x=w694) -> (x+1=w695:i32)
                                n623 = local write "Aktueller Messschritt"(w695) -> ()
                                }
                                frame #1 {
                                n624 = local read "# Photosignale"() -> (w705:i32)
                                n625 = local read "# Bilder/Messschritt"() -> (w701:i32)
                                n626 = local read "Detektionskamera"() -> (w704:T4)
                                n627 = local read "Einzelbilder speichern"() -> (w699:bool)
                                n628 = for {
                                N: w705 -> [_]
                                n629 = Wait (ms)(milliseconds to wait=u32 10 ("Zu wartende ms")) -> ()  [unwired: 1 out]
                                n630 = local read "LAPD-Kanal (Meilhaus)"() -> (w723:u32)
                                n631 = local read "LAPD Spannung (V)"() -> (w721:dbl)
                                n632 = call "AISingle.vi"("Time Out"=u32 0, "Channel Number"=w723, "Board Number"=u32 0) -> ("Analog Input Voltage"=w722:dbl)
                                n633 = Add(x=w722, y=w721) -> (x+y=w720:dbl)
                                n634 = local write "LAPD Spannung (V)"(w720) -> ()
                                }
                                n635 = call "camera_acquisition_sequence.vi"("Session In"=w704, "Desired image number"=w701) -> ("Image Array"=w698:T3[], "error out"=w703:errorcluster)  [unwired: 2 in, 1 out]
                                n636 = case shown="True" w699 {
                                tunnel: w703 -> [w707 w715]
                                tunnel: [w707 w714] -> w702
                                tunnel: w701 -> [w706 w713]
                                tunnel: [w706 w713] -> w700
                                tunnel: w698 -> [_ w712]
                                frame #0 {
                                }
                                frame #1 {
                                n637 = local read "Aktueller Messschritt"() -> (w718:i32)
                                n638 = local read "Save folder"() -> (w710:string)
                                n639 = Concatenate Strings(w710, "Einzelbilder\\" ("String")) -> (w708:string)
                                n640 = Format Into String(format string="%05.0f" ("Format-String"), initial string="#" ("Eingangs-String"), w718) -> (resulting string=w711:string)  [unwired: 1 in, 1 out]
                                n641 = call "save images.vi"("Save Folder"=w708, "File name prefix"=w711, "Array"=w712, "error out 2"=w715, "Bilder/Messschritt"=w713) -> ("error out"=w714:errorcluster)
                                }
                                }
                                n642 = for {
                                N: w700 -> [_]
                                tunnel: w702 -> [w731]
                                tunnel: w698 -> [w729] mode=indexing
                                n643 = call "IMAQ ImageToArray"("error in (no error)"=w731, "Image"=w729) -> ("error out"=w730:errorcluster, "Image Pixels (U8)"=w728:u8[][])  [unwired: 2 in, 3 out]
                                n644 = local read "Gemitteltes Bild"() -> (w726:u64[][])
                                n645 = To Unsigned Quad Integer(1:w728) -> (0:w733:u64[][])
                                n646 = local write "Fehler (Ausgang)"(w730) -> ()
                                n647 = local read "Summierte Helligkeit (a.u.)"() -> (w734:u64)
                                n648 = Add Array Elements(numeric array=w733) -> (sum=w732:u64)
                                n649 = Add(x=w726, y=w728) -> (x+y=w727:u64[][])
                                n650 = local write "Gemitteltes Bild"(w727) -> ()
                                n651 = Add(x=w732, y=w734) -> (x+y=w735:u64)
                                n652 = local write "Summierte Helligkeit (a.u.)"(w735) -> ()
                                }
                                }
                                frame #2 {
                                n653 = local read "Rasterart"() -> (w745:T2)
                                n654 = case shown="\"Linescan(z)\"" w745 {
                                tunnel: [w767 w768 w770 w771] -> w744
                                tunnel: [w766 w769 w770 w771] -> w743
                                frame #0 {
                                n655 = local read "Current x step"() -> (w767:i32)
                                n656 = local read "Current y step"() -> (w766:i32)
                                }
                                frame #1 {
                                n657 = local read "Current z step"() -> (w768:i32)
                                n658 = local read "Current y step"() -> (w769:i32)
                                }
                                frame #2 {
                                n659 = local read "Current z step"() -> (w770:i32)
                                }
                                frame #3 {
                                n660 = local read "Current x step"() -> (w771:i32)
                                }
                                }
                                n661 = local read "# Bilder/Messschritt"() -> (w740:i32)
                                n662 = local read "Gemitteltes Bild"() -> (w742:u64[][])
                                n663 = local read "2D-Intensitätsverteilung (MCP)"() -> (w747:dbl[][])
                                n664 = local read "2D-Intensitätsverteilung (LAPD)"() -> (w746:dbl[][])
                                n665 = local read "LAPD Spannung (V)"() -> (w751:dbl)
                                n666 = local read "Summierte Helligkeit (a.u.)"() -> (w752:u64)
                                n667 = local read "Gemittelte Bilder speichern"() -> (w736:bool)
                                n668 = local read "# Photosignale"() -> (w750:i32)
                                n669 = local read "Image Display"() -> (w738:T3)
                                n670 = Divide(x=w742, y=w740) -> (x/y=w741:dbl[][])
                                n671 = Divide(x=w751, y=w750) -> (x/y=w748:dbl)
                                n672 = call "IMAQ ArrayToImage"("Image Pixels (U8)"=w741, "Image"=w738) -> ("Image Out"=w739:T3)  [unwired: 8 in, 1 out]
                                n673 = Replace Array Subset(array=w746, new element=w748, index (row)=w744, index (col)=w743) -> (w749:dbl[][])
                                n674 = local write "LAPD Spannung (V)"(w748) -> ()
                                n675 = Replace Array Subset(array=w747, new element=w752, index (row)=w744, index (col)=w743) -> (w753:dbl[][])
                                n676 = case shown="True" w736 {
                                tunnel: w739 -> [w754 w765]
                                tunnel: [w754 w756] -> w737
                                frame #0 {
                                }
                                frame #1 {
                                n677 = local read "Aktueller Messschritt"() -> (w760:i32)
                                n678 = local read "Save folder"() -> (w762:string)
                                n679 = Format Into String(format string="%05.0f" ("Format-String"), initial string="#" ("Eingangs-String"), w760) -> (resulting string=w759:string)  [unwired: 1 in, 1 out]
                                n680 = Concatenate Strings(w762, "Gemittelte Bilder\\" ("String"), w759, ".png" ("String")) -> (w758:string)
                                n681 = String To Path(string=w758) -> (path=w757:path)
                                n682 = call-poly "IMAQ Write File 2"("File Path"=w757, "Image"=w765) -> ("Image Out (duplicate)"=w756:T3)  [unwired: 8 in, 1 out]
                                }
                                }
                                n683 = local write "2D-Intensitätsverteilung (LAPD)"(w749) -> ()
                                n684 = local write "2D-Intensitätsverteilung (MCP)"(w753) -> ()
                                n685 = local write "Image Display"(w737) -> ()
                                }
                                }
                                }
                                frame #1 {
                                n686 = local read "Rasterschritt [µm]"() -> (w781:dbl[])
                                n687 = local read "y-Achse"() -> (w777:i32)
                                n688 = Decrement(x=w777) -> (x-1=w780:i32)
                                n689 = Index Array(array=w781, index=w780) -> (element=w776:dbl)
                                n690 = local read "Aktueller Messschritt"() -> (w774:i32)
                                n691 = local read "Start time [ms]"() -> (w775:timestamp)
                                n692 = local read "# Messschritte"() -> (w773:i32)
                                n693 = Not Equal?(x=w776, y=0.0) -> (x != y?=w778:bool)
                                n694 = case shown="True" w778 {
                                tunnel: w777 -> [_ w783]
                                tunnel: w776 -> [_ w782]
                                frame #0 {
                                }
                                frame #1 {
                                # "Fahre nächste y-Position an"
                                n695 = call "stage_move_axis_relative.vi"("Achse"=w783, "Schrittweite [µm]"=w782) -> ("error out"=w785:errorcluster, "xyz-Position OUT [mm]"=w784:dbl[])  [unwired: 1 in, 1 out]
                                n696 = local write "Aktuelle xyz-Position [mm]"(w784) -> ()
                                n697 = local write "Fehler (Ausgang)"(w785) -> ()
                                }
                                }
                                n698 = call "estimate_stopp_time.vi"("Aktueller Messschritt"=w774, "# Messschritte"=w773, "Startzeit"=w775) -> ("Stopp Zeit"=w772:string)  [unwired: 8 in]
                                n699 = local write "Geschätzte Messzeit"(w772) -> ()
                                }
                              }
                              n700 = local read "y-Achse"() -> (w677:i32)
                              n701 = local read "# Rasterschritte"() -> (w683:i32[])
                              n702 = Decrement(x=w677) -> (x-1=w679:i32)
                              n703 = local read "Rasterung ON/OFF"() -> (w685:bool)
                              n704 = Increment(x=w678) -> (x+1=w680:i32)
                              n705 = Index Array(array=w683, index=w679) -> (element=w682:i32)
                              n706 = Equal?(x=w682, y=w680) -> (x = y?=w681:bool)
                              n707 = Not(x=w685) -> (.not. x?=w686:bool)
                              n708 = Or(x=w681, y=w686) -> (x .or. y?=w684:bool)
                              "Current y step" <- w678
                            }
                          }
                          frame #1 {
                            n709 = flat-sequence {
                              frame #0 {
                                n710 = local read "Rasterschritt [µm]"() -> (w792:dbl[])
                                n711 = local read "y-Achse"() -> (w787:i32)
                                n712 = Decrement(x=w787) -> (x-1=w791:i32)
                                n713 = local read "Start xyz-Position [mm]"() -> (w786:dbl[])
                                n714 = Index Array(array=w792, index=w791) -> (element=w790:dbl)
                                n715 = Not Equal?(x=w790, y=0.0) -> (x != y?=w788:bool)
                                n716 = case shown="True" w788 {
                                tunnel: w787 -> [_ w794]
                                tunnel: w786 -> [_ w793]
                                frame #0 {
                                }
                                frame #1 {
                                # "Fahre Startposition für y an"
                                n717 = call "stage_move_axis_absolute.vi"("Ziel xyz IN [mm]"=w793, "Achse"=w794) -> ("error out"=w796:errorcluster, "Ziel xyz OUT [mm]"=w795:dbl[])  [unwired: 1 in, 1 out]
                                n718 = local write "Aktuelle xyz-Position [mm]"(w795) -> ()
                                n719 = local write "Fehler (Ausgang)"(w796) -> ()
                                }
                                }
                              }
                              frame #1 {
                                n720 = local read "Rasterschritt [µm]"() -> (w802:dbl[])
                                n721 = local read "x-Achse"() -> (w797:i32)
                                n722 = Decrement(x=w797) -> (x-1=w798:i32)
                                n723 = Index Array(array=w802, index=w798) -> (element=w799:dbl)
                                n724 = Not Equal?(x=w799, y=0.0) -> (x != y?=w800:bool)
                                n725 = case shown="True" w800 {
                                tunnel: w799 -> [_ w804]
                                tunnel: w797 -> [_ w803]
                                frame #0 {
                                }
                                frame #1 {
                                # "Fahre nächste Position für x an"
                                n726 = call "stage_move_axis_relative.vi"("Achse"=w803, "Schrittweite [µm]"=w804) -> ("error out"=w805:errorcluster, "xyz-Position OUT [mm]"=w806:dbl[])  [unwired: 1 in, 1 out]
                                n727 = local write "Aktuelle xyz-Position [mm]"(w806) -> ()
                                n728 = local write "Fehler (Ausgang)"(w805) -> ()
                                }
                                }
                              }
                            }
                          }
                        }
                        n729 = local read "# Rasterschritte"() -> (w672:i32[])
                        n730 = local read "x-Achse"() -> (w668:i32)
                        n731 = Decrement(x=w668) -> (x-1=w676:i32)
                        n732 = local read "Rasterung ON/OFF"() -> (w671:bool)
                        n733 = Increment(x=w667) -> (x+1=w675:i32)
                        n734 = Index Array(array=w672, index=w676) -> (element=w673:i32)
                        n735 = Equal?(x=w673, y=w675) -> (x = y?=w674:bool)
                        n736 = Not(x=w671) -> (.not. x?=w670:bool)
                        n737 = Or(x=w674, y=w670) -> (x .or. y?=w669:bool)
                        "Current x step" <- w667
                      }
                    }
                    frame #1 {
                      n738 = flat-sequence {
                        frame #0 {
                          n739 = local read "Rasterschritt [µm]"() -> (w810:dbl[])
                          n740 = local read "x-Achse"() -> (w807:i32)
                          n741 = Decrement(x=w807) -> (x-1=w811:i32)
                          n742 = local read "Start xyz-Position [mm]"() -> (w808:dbl[])
                          n743 = Index Array(array=w810, index=w811) -> (element=w812:dbl)
                          n744 = Not Equal?(x=w812, y=0.0) -> (x != y?=w809:bool)
                          n745 = case shown="True" w809 {
                            tunnel: w808 -> [_ w815]
                            tunnel: w807 -> [_ w814]
                            frame #0 {
                            }
                            frame #1 {
                              # "Fahre Startposition für x an"
                              n746 = call "stage_move_axis_absolute.vi"("Ziel xyz IN [mm]"=w815, "Achse"=w814) -> ("error out"=w816:errorcluster, "Ziel xyz OUT [mm]"=w817:dbl[])  [unwired: 1 in, 1 out]
                              n747 = local write "Aktuelle xyz-Position [mm]"(w817) -> ()
                              n748 = local write "Fehler (Ausgang)"(w816) -> ()
                            }
                          }
                        }
                        frame #1 {
                          n749 = local read "Rasterschritt [µm]"() -> (w823:dbl[])
                          n750 = local read "z-Achse"() -> (w818:i32)
                          n751 = Decrement(x=w818) -> (x-1=w822:i32)
                          n752 = Index Array(array=w823, index=w822) -> (element=w821:dbl)
                          n753 = Not Equal?(x=w821, y=0.0) -> (x != y?=w819:bool)
                          n754 = case shown="True" w819 {
                            tunnel: w821 -> [_ w826]
                            tunnel: w818 -> [_ w824]
                            frame #0 {
                            }
                            frame #1 {
                              # "Fahre nächste Position für z an"
                              n755 = call "stage_move_axis_relative.vi"("Achse"=w824, "Schrittweite [µm]"=w826) -> ("error out"=w827:errorcluster, "xyz-Position OUT [mm]"=w825:dbl[])  [unwired: 1 in, 1 out]
                              n756 = local write "Aktuelle xyz-Position [mm]"(w825) -> ()
                              n757 = local write "Fehler (Ausgang)"(w827) -> ()
                            }
                          }
                        }
                      }
                    }
                  }
                  n758 = local read "# Rasterschritte"() -> (w664:i32[])
                  n759 = local read "z-Achse"() -> (w657:i32)
                  n760 = local read "Rasterung ON/OFF"() -> (w665:bool)
                  n761 = Decrement(x=w657) -> (x-1=w660:i32)
                  n762 = Increment(x=w658) -> (x+1=w661:i32)
                  n763 = Index Array(array=w664, index=w660) -> (element=w663:i32)
                  n764 = Equal?(x=w663, y=w661) -> (x = y?=w662:bool)
                  n765 = Not(x=w665) -> (.not. x?=w666:bool)
                  n766 = Or(x=w662, y=w666) -> (x .or. y?=w659:bool)
                  "Current z step" <- w658
                }
              }
              frame #1 {
                n767 = local read "Summierte Helligkeit speichern"() -> (w842:bool)
                n768 = local read "LAPD-Daten speichern"() -> (w841:bool)
                n769 = local read "Summierte Helligkeit speichern"() -> (w830:bool)
                n770 = flat-sequence {
                  frame #0 {
                    # "Zur Ausgangsposition zurückfahren"
                    n771 = local read "Start xyz-Position [mm]"() -> (w908:dbl[])
                    n772 = local read "Detektionskamera"() -> (w898:T4)
                    n773 = local read "Buffer Interval"() -> (w897:u32)
                    n774 = call "camera_create_configuration.vi"("BufferInterval"=w897, "Session Out 2"=w898) -> ("Fehler (Ausgang)"=w896:errorcluster, "Ereignisregistrierung (Referenz)"=w899:refnum<event-registration>)  [unwired: 1 in, 1 out]
                    n775 = local write "Ereignis: FrameDone?"(w899) -> ()
                    n776 = local read "x-Achse"() -> (w905:i32)
                    n777 = call "stage_move_axis_absolute.vi"("error in"=w896, "Ziel xyz IN [mm]"=w908, "Achse"=w905) -> ("error out"=w901:errorcluster)  [unwired: 2 out]
                    n778 = local read "y-Achse"() -> (w906:i32)
                    n779 = call "stage_move_axis_absolute.vi"("error in"=w901, "Ziel xyz IN [mm]"=w908, "Achse"=w906) -> ("error out"=w902:errorcluster)  [unwired: 2 out]
                    n780 = local read "z-Achse"() -> (w907:i32)
                    n781 = call "stage_move_axis_absolute.vi"("error in"=w902, "Ziel xyz IN [mm]"=w908, "Achse"=w907) -> ("error out"=w903:errorcluster, "Fertig?"=w904:bool, "Ziel xyz OUT [mm]"=w909:dbl[])
                    n782 = Not(x=w904) -> (.not. x?=w900:bool)
                    n783 = local write "Aktuelle xyz-Position [mm]"(w909) -> ()
                    n784 = local write "Fehler (Ausgang)"(w903) -> ()
                    n785 = local write "Rasterung ON/OFF"(w900) -> ()
                    n786 = local write "Rasterung läuft"(w900) -> ()
                  }
                }
                n787 = local read "Gemittelte Bilder speichern"() -> (w831:bool)
                n788 = local read "2D-Intensitätsverteilung (MCP)"() -> (w840:dbl[][])
                n789 = local read "2D-Intensitätsverteilung (LAPD)"() -> (w836:dbl[][])
                n790 = local read "LAPD-Daten speichern"() -> (w829:bool)
                n791 = local read "Einzelbilder speichern"() -> (w828:bool)
                n792 = control-ref of="2D-Intensitätsverteilung (MCP)"() -> (w839:refnum<vi>)
                n793 = control-ref of="2D-Intensitätsverteilung (LAPD)"() -> (w833:refnum<vi>)
                n794 = case shown="True" w841 {
                  frame #0 {
                  }
                  frame #1 {
                    n795 = local read "Save folder"() -> (w914:string)
                    n796 = local read "2D-Intensitätsverteilung (LAPD)"() -> (w912:dbl[][])
                    n797 = Concatenate Strings(w914, "\\" ("String"), "2D_Intensitaetsverteilung_LAPD.dat" ("String")) -> (w916:string)
                    n798 = String To Path(string=w916) -> (path=w915:path)
                    n799 = call-poly <vilib>:"Write To Spreadsheet File.vi"("format (%.3f)"="%.;%.5f", "2D data"=w912, "file path (dialog if empty)"=w915) -> ()  [unwired: 5 in, 1 out]
                  }
                }
                n800 = Compound Arithmetic op=OR(w828, w829, w831, w830) -> (w832:bool)
                n801 = case shown="True" w842 {
                  frame #0 {
                  }
                  frame #1 {
                    n802 = local read "Save folder"() -> (w920:string)
                    n803 = local read "2D-Intensitätsverteilung (MCP)"() -> (w922:dbl[][])
                    n804 = Concatenate Strings(w920, "\\" ("String"), "2D_Intensitaetsverteilung_MCP.dat" ("String")) -> (w918:string)
                    n805 = String To Path(string=w918) -> (path=w919:path)
                    n806 = call-poly <vilib>:"Write To Spreadsheet File.vi"("format (%.3f)"="%.;%8.0f", "2D data"=w922, "file path (dialog if empty)"=w919) -> ()  [unwired: 5 in, 1 out]
                  }
                }
                n807 = case shown="True" w832 {
                  frame #0 {
                  }
                  frame #1 {
                    n808 = local read "Rasterschritt [µm]"() -> (w844:dbl[])
                    n809 = local read "Start xyz-Position [mm]"() -> (w847:dbl[])
                    n810 = local read "# Rasterschritte"() -> (w848:i32[])
                    n811 = local read "Save folder"() -> (w846:string)
                    n812 = Divide(x=w844, y=1000) -> (x/y=w845:dbl[])
                    n813 = local read "Rasterart"() -> (w849:T2)
                    n814 = case shown="\"2D-Scan(yz)\"" w849 {
                      tunnel: w848 -> [w852 w859 w871 w892]
                      tunnel: w847 -> [w850 w861 w869 w893]
                      tunnel: w846 -> [w853 w862 w868 w891]
                      tunnel: w845 -> [w851 w860 w870 w882]
                      frame #0 {
                        w858 = 0 ("Index")
                        n815 = Index Array(array=w850, index=w858) -> (element=w856:dbl)
                        n816 = Index Array(array=w851, index=w858) -> (element=w854:dbl)
                        n817 = Index Array(array=w852, index=w858) -> (element=w855:i32)
                        n818 = call "create_axis_vector_file.vi"("Save folder"=w853, "Dateiname"="xAchse.dat", "Start"=w856, "Schrittlänge"=w854, "# Schritte"=w855) -> ()  [unwired: 11 in]
                      }
                      frame #1 {
                        w867 = 2 ("Index")
                        n819 = Index Array(array=w861, index=w867) -> (element=w865:dbl)
                        n820 = Index Array(array=w860, index=w867) -> (element=w863:dbl)
                        n821 = Index Array(array=w859, index=w867) -> (element=w864:i32)
                        n822 = call "create_axis_vector_file.vi"("Save folder"=w862, "Dateiname"="xAchse.dat", "Start"=w865, "Schrittlänge"=w863, "# Schritte"=w864) -> ()  [unwired: 11 in]
                      }
                      frame #2 {
                        w880 = 1 ("Index")
                        w881 = 0 ("Index")
                        n823 = Index Array(array=w869, index #1=w881, index #2=w880) -> (element #1=w877:dbl, element #2=w874:dbl)
                        n824 = Index Array(array=w870, index #1=w881, index #2=w880) -> (element #1=w875:dbl, element #2=w873:dbl)
                        n825 = Index Array(array=w871, index #1=w881, index #2=w880) -> (element #1=w876:i32, element #2=w872:i32)
                        n826 = call "create_axis_vector_file.vi"("Save folder"=w868, "Dateiname"="yAchse.dat", "Start"=w874, "Schrittlänge"=w873, "# Schritte"=w872) -> ()  [unwired: 11 in]
                        n827 = call "create_axis_vector_file.vi"("Save folder"=w868, "Dateiname"="xAchse.dat", "Start"=w877, "Schrittlänge"=w875, "# Schritte"=w876) -> ()  [unwired: 11 in]
                      }
                      frame #3 {
                        w894 = 2 ("Index")
                        w895 = 1 ("Index")
                        n828 = Index Array(array=w893, index #1=w895, index #2=w894) -> (element #1=w888:dbl, element #2=w885:dbl)
                        n829 = Index Array(array=w882, index #1=w895, index #2=w894) -> (element #1=w886:dbl, element #2=w884:dbl)
                        n830 = Index Array(array=w892, index #1=w895, index #2=w894) -> (element #1=w887:i32, element #2=w883:i32)
                        n831 = call "create_axis_vector_file.vi"("Save folder"=w891, "Dateiname"="xAchse.dat", "Start"=w885, "Schrittlänge"=w884, "# Schritte"=w883) -> ()  [unwired: 11 in]
                        n832 = call "create_axis_vector_file.vi"("Save folder"=w891, "Dateiname"="yAchse.dat", "Start"=w888, "Schrittlänge"=w886, "# Schritte"=w887) -> ()  [unwired: 11 in]
                      }
                    }
                  }
                }
                n833 = Array Max & Min(array=w836) -> (max value=w835:dbl, min value=w834:dbl)  [unwired: 2 out]
                n834 = Array Max & Min(array=w840) -> (max value=w838:dbl, min value=w837:dbl)  [unwired: 2 out]
                n835 = property class="IntGraph (strikt)"(reference=w833, "ZScale.Maximum"=w835, "ZScale.Minimum"=w834) -> ()  [unwired: 1 in, 2 out]
                n836 = property class="IntGraph (strikt)"(reference=w839, "ZScale.Maximum"=w838, "ZScale.Minimum"=w837) -> ()  [unwired: 1 in, 2 out]
              }
            }
          }
          event #4 {
            n837 = event-data() -> ("NewVal"=w926:bool)  [unwired: 1 in]
            n838 = local read "Kamera"() -> (w927:bool)
            n839 = local read "HV-Steuerung"() -> (w924:bool)
            n840 = Compound Arithmetic op=AND(w927, w926, w924) -> (w925:bool)
            n841 = case shown="True" w925 {
              frame #0 {
                n842 = local write "Spannungsscan läuft"(FALSE ("Messung läuft")) -> ()
              }
              frame #1 {
                n843 = stacked-sequence {
                  frame #0 {
                    n844 = flat-sequence {
                      tunnel: [w942] -> w929
                      tunnel: w929 -> [w958]
                      frame #0 {
                        n845 = control-ref of="Shutter time (ms)"() -> (w955:refnum<vi>)
                        n846 = local read "Suppressor-Spannung [V]"() -> (w932:dbl)
                        n847 = property class="Ring (strikt)"(reference=w955) -> ("RingText.Text"=w954:string)  [unwired: 1 in, 2 out]
                        n848 = local read "# Bilder/Messschritt"() -> (w948:i32)
                        n849 = local read "Spannungsstart [V]"() -> (w936:dbl[])
                        n850 = local read "# Spannungsschritte"() -> (w951:i32[])
                        n851 = local read "Spannungsweite [V]"() -> (w950:dbl[])
                        n852 = local read "Tip-Spannung [V]"() -> (w933:dbl)
                        n853 = local read "P-Schirm-Spannung [V]"() -> (w940:dbl)
                        n854 = local write "Aktueller Messschritt"(0 ("Aktueller Messschritt")) -> ()
                        n855 = local read "MCP-Spannung [V]"() -> (w939:dbl)
                        n856 = local read "Leistung (iK) [mW]"() -> (w938:dbl)
                        n857 = local read "Polarisation [°]"() -> (w945:dbl)
                        n858 = local read "Messlogbuch"() -> (w947:path)
                        n859 = Decimal String To Number(string=w954) -> (number=w937:i32)  [unwired: 2 in, 1 out]
                        n860 = local read "Proben-ID"() -> (w946:string)
                        n861 = Multiply(x=w948, y=w937) -> (x*y=w949:i32)
                        n862 = Divide(x=w950, y=w951) -> (x/y=w952:dbl[])
                        n863 = local read "ROI"() -> (w943:i32[])
                        n864 = Replace Array Subset(array=w936, new element #1=w933, index #1=0 ("Index"), new element #2=w932, index #2=1 ("Index")) -> (w931:dbl[])
                        n865 = local write "Spannungsschritt [V]"(w952) -> ()
                        n866 = Get Date/Time In Seconds() -> (seconds since 1Jan1904=w930:timestamp)
                        n867 = local write "Aktuelle Spannung [V]"(w931) -> ()
                        n868 = call "stage_get_current_xyz.vi"() -> ("Aktuelle xyz-Position OUT [mm]"=w941:dbl[])  [unwired: 3 in, 1 out]
                        n869 = call "create_measure_log_entry.vi"("Messlogbuch-Pfad"=w947, "Probe"=w946, "Polarisation [°]"=w945, "Messart"="Spannungsscan", "ROI"=w943, "Messungen/Messschritt"=w948, "Maximalleistung (iK) [mW]"=w938, "Tip-Spannung [V]"=w933, "Suppressor-Spannung [V]"=w932, "Zeit/Messschritt [ms]"=w937, "MCP-Spannung [V]"=w939, "Zeit/Messung [ms]"=w949, "Phosphorschirm-Spannung [V]"=w940, "xyz [mm]"=w941) -> ("Messung Nr."=w942:i32)  [unwired: 4 in, 1 out]
                        n870 = local write "Start time [ms]"(w930) -> ()
                        n871 = local write "Spannungsstart [V]"(w931) -> ()
                      }
                      frame #1 {
                        n872 = local read "Day folder"() -> (w964:string)
                        n873 = local read "Fehler (Ausgang)"() -> (w959:errorcluster)
                        n874 = local read "# Spannungsschritte"() -> (w973:i32[])
                        n875 = local read "Einzelbilder speichern"() -> (w966:bool)
                        n876 = call "create_save_folder.vi"("Day folder"=w964, "Measuring number"=w958, "Measuring folder"="Spannungsscan" ("Subfolder"), "error in"=w959) -> ("Save Folder"=w963:string, "Error Out"=w962:errorcluster)  [unwired: 5 in]
                        n877 = local write "Save folder"(w963) -> ()
                        n878 = Index Array(array=w973, index #1=0 ("Index"), index #2=1 ("Index")) -> (element #1=w970:i32, element #2=w969:i32)
                        n879 = local read "Gemittelte Bilder speichern"() -> (w967:bool)
                        n880 = Multiply(x=w970, y=w969) -> (x*y=w956:i32)
                        n881 = case shown="True" w966 {
                          tunnel: w962 -> [w974 w976]
                          tunnel: [w974 w975] -> w961
                          frame #0 {
                          }
                          frame #1 {
                            n882 = local read "Save folder"() -> (w979:string)
                            n883 = Concatenate Strings(w979, "\\Einzelbilder" ("Subfolder")) -> (w977:string)
                            n884 = String To Path(string=w977) -> (path=w980:path)
                            n885 = call <vilib>:"Check if File or Folder Exists.vi"("error in (no error)"=w976, "path"=w980) -> ("error out"=w975:errorcluster, "file or folder exists?"=w981:bool, "dup path"=w982:path)  [unwired: 7 in]
                            n886 = case shown="False" w981 {
                              tunnel: w982 -> [w983 _]
                              frame #0 {
                                n887 = Create Folder(path (use dialog)=w983) -> ()  [unwired: 2 in, 3 out]
                              }
                              frame #1 {
                              }
                            }
                          }
                        }
                        n888 = local read "Kamera"() -> (w968:bool)
                        n889 = local write "# Messschritte"(w956) -> ()
                        n890 = case shown="True" w967 {
                          tunnel: w961 -> [w984 w986]
                          tunnel: [w984 w985] -> w960
                          frame #0 {
                          }
                          frame #1 {
                            n891 = local read "Save folder"() -> (w990:string)
                            n892 = Concatenate Strings(w990, "\\Gemittelte Bilder" ("Subfolder")) -> (w992:string)
                            n893 = String To Path(string=w992) -> (path=w989:path)
                            n894 = call <vilib>:"Check if File or Folder Exists.vi"("error in (no error)"=w986, "path"=w989) -> ("error out"=w985:errorcluster, "file or folder exists?"=w988:bool, "dup path"=w987:path)  [unwired: 7 in]
                            n895 = case shown="False" w988 {
                              tunnel: w987 -> [w993 _]
                              frame #0 {
                                n896 = Create Folder(path (use dialog)=w993) -> ()  [unwired: 2 in, 3 out]
                              }
                              frame #1 {
                              }
                            }
                          }
                        }
                        n897 = case shown="True" w968 {
                          tunnel: [w994 w996] -> w957
                          tunnel: w960 -> [w994 w995]
                          frame #0 {
                          }
                          frame #1 {
                            n898 = local read "Ereignis: FrameDone?"() -> (w997:refnum<event-registration>)
                            n899 = local read "Detektionskamera"() -> (w998:T4)
                            n900 = call "camera_release_configuration.vi"("error in"=w995, "Session In"=w998, "Ereignisregistrierung (Referenz) 2"=w997) -> ("error out"=w996:errorcluster)  [unwired: 1 out]
                          }
                        }
                        n901 = local write "Fehler (Ausgang)"(w957) -> ()
                      }
                    }
                  }
                  frame #1 {
                    n902 = flat-sequence {
                      frame #0 {
                        w1004 = 1 ("Index")
                        w1005 = 0 ("Index")
                        n903 = local read "Spannungsstart [V]"() -> (w1000:dbl[])
                        n904 = local read "# Spannungsschritte"() -> (w1015:i32[])
                        n905 = local read "Spannungsschritt [V]"() -> (w1003:dbl[])
                        n906 = Index Array(array=w1015, index #1=w1005, index #2=w1004) -> (element #1=w1013:i32, element #2=w1014:i32)
                        n907 = control-ref of="2D-Intensitätsverteilung (MCP)"() -> (w999:refnum<vi>)
                        n908 = Initialize Array(0.0 ("y"), w1013, w1014) -> (w1011:dbl[][])
                        n909 = Index Array(array=w1003, index #1=w1005, index #2=w1004) -> (element #1=w1007:dbl, element #2=w1006:dbl)
                        n910 = Index Array(array=w1000, index #1=w1005, index #2=w1004) -> (element #1=w1002:dbl, element #2=w1001:dbl)
                        n911 = local write "2D-Intensitätsverteilung (MCP)"(w1011) -> ()
                        n912 = property class="IntGraph (strikt)"(reference=w999, "XScale.Offset"=w1002, "XScale.Multiplier"=w1007, "YScale.Offset"=w1001, "YScale.Multiplier"=w1006, "XScale.MinorInc"=w1007, "YScale.MinorInc"=w1006, "XScale.NameLbl.Text"="Tip-Spannung [V]" ("Y-Achse.Namensbeschriftung.Text"), "YScale.NameLbl.Text"="Suppressor-Spannung [V]" ("X-Achse.Namensbeschriftung.Text")) -> (error out=w1010:errorcluster)  [unwired: 1 in, 1 out]
                        n913 = local write "Fehler (Ausgang)"(w1010) -> ()
                      }
                      frame #1 {
                        n914 = local write "Spannungsscan läuft"(TRUE ("Messung läuft")) -> ()
                      }
                    }
                  }
                }
              }
            }
          }
          event #5 {
            n915 = event-data() -> ("NewVal"=w1019:bool)  [unwired: 1 in]
            n916 = local read "Kamera"() -> (w1020:bool)
            n917 = local read "HV-Steuerung"() -> (w1017:bool)
            n918 = Compound Arithmetic op=AND(w1020, w1019, w1017) -> (w1018:bool)
            n919 = case shown="True" w1018 {
              frame #0 {
                n920 = local write "x-U-Scan läuft"(FALSE ("Messung läuft")) -> ()
              }
              frame #1 {
                n921 = stacked-sequence {
                  frame #0 {
                    n922 = flat-sequence {
                      tunnel: [w1035] -> w1022
                      tunnel: w1022 -> [w1061]
                      frame #0 {
                        n923 = local read "Raum-Koordinate"() -> (w1027:enum16{"x-Achse", "y-Achse", "z-Achse"})
                        n924 = local read "# x-U-Scan Spannungsschritte"() -> (w1050:i32)
                        n925 = local read "x-U-Scan Spannungsweite [V]"() -> (w1049:dbl)
                        n926 = local read "# x-U-Scan Rasterschritte"() -> (w1047:i32)
                        n927 = local read "# Bilder/Messschritt"() -> (w1036:i32)
                        n928 = local read "x-U-Scan Rasterweite [µm]"() -> (w1048:dbl)
                        n929 = call "stage_get_current_xyz.vi"() -> ("Aktuelle xyz-Position OUT [mm]"=w1031:dbl[])  [unwired: 3 in, 1 out]
                        n930 = local read "ROI"() -> (w1039:i32[])
                        n931 = Add(x=w1027, y=1) -> (x+y=w1025:i32)
                        n932 = local write "Start xyz-Position [mm]"(w1031) -> ()
                        n933 = Index Array(array=w1031, index=w1027) -> (element=w1030:dbl)
                        n934 = local write "Aktueller Messschritt"(0 ("Aktueller Messschritt")) -> ()
                        n935 = local write "Achs-ID"(w1025) -> ()
                        n936 = control-ref of="Shutter time (ms)"() -> (w1054:refnum<vi>)
                        n937 = local write "x-U-Scan Startposition [mm]"(w1030) -> ()
                        n938 = local read "Spannungs-Koordinate"() -> (w1045:enum16{"Tip-Spannung", "Suppressor-Spannung"})
                        n939 = property class="Ring (strikt)"(reference=w1054) -> ("RingText.Text"=w1053:string)  [unwired: 1 in, 2 out]
                        n940 = local read "Tip-Spannung [V]"() -> (w1028:dbl)
                        n941 = Divide(x=w1048, y=w1047) -> (x/y=w1046:dbl)
                        n942 = Divide(x=w1049, y=w1050) -> (x/y=w1051:dbl)
                        n943 = local read "P-Schirm-Spannung [V]"() -> (w1034:dbl)
                        n944 = local write "x-U-Scan Spannungsschritt [V]"(w1051) -> ()
                        n945 = Decimal String To Number(string=w1053) -> (number=w1037:i32)  [unwired: 2 in, 1 out]
                        n946 = local write "x-U-Scan Rasterschritt [µm]"(w1046) -> ()
                        n947 = local read "MCP-Spannung [V]"() -> (w1033:dbl)
                        n948 = case shown="\"Suppressor-Spannung\"" w1045 {
                          tunnel: [refnum<k21> "Dev0/Ao1" ("Spannungskanal") refnum<k21> "Dev0/Ao0" ("Spannungskanal")] -> w1044
                          tunnel: [w1055 w1057] -> w1024
                          frame #0 {
                            n949 = local read "Tip-Spannung [V]"() -> (w1055:dbl)
                          }
                          frame #1 {
                            n950 = local read "Suppressor-Spannung [V]"() -> (w1057:dbl)
                          }
                        }
                        n951 = local read "Leistung (iK) [mW]"() -> (w1032:dbl)
                        n952 = local read "Polarisation [°]"() -> (w1041:dbl)
                        n953 = Get Date/Time In Seconds() -> (seconds since 1Jan1904=w1023:timestamp)
                        n954 = local read "Messlogbuch"() -> (w1043:path)
                        n955 = local read "Proben-ID"() -> (w1042:string)
                        n956 = local read "Suppressor-Spannung [V]"() -> (w1029:dbl)
                        n957 = Multiply(x=w1036, y=w1037) -> (x*y=w1038:i32)
                        n958 = local write "Start time [ms]"(w1023) -> ()
                        n959 = local write "Spannungskanal"(w1044) -> ()
                        n960 = local write "x-U-Scan aktuelle Spannung [V]"(w1024) -> ()
                        n961 = local write "x-U-Scan Spannungsstart [V]"(w1024) -> ()
                        n962 = call "create_measure_log_entry.vi"("Messlogbuch-Pfad"=w1043, "Probe"=w1042, "Polarisation [°]"=w1041, "Messart"="x-U-Scan", "ROI"=w1039, "Messungen/Messschritt"=w1036, "Maximalleistung (iK) [mW]"=w1032, "Tip-Spannung [V]"=w1028, "Suppressor-Spannung [V]"=w1029, "Zeit/Messschritt [ms]"=w1037, "MCP-Spannung [V]"=w1033, "Zeit/Messung [ms]"=w1038, "Phosphorschirm-Spannung [V]"=w1034, "xyz [mm]"=w1031) -> ("Messung Nr."=w1035:i32)  [unwired: 4 in, 1 out]
                      }
                      frame #1 {
                        n963 = local read "Day folder"() -> (w1069:string)
                        n964 = local read "Fehler (Ausgang)"() -> (w1064:errorcluster)
                        n965 = local read "Einzelbilder speichern"() -> (w1071:bool)
                        n966 = local read "# x-U-Scan Spannungsschritte"() -> (w1060:i32)
                        n967 = local read "# x-U-Scan Rasterschritte"() -> (w1059:i32)
                        n968 = call "create_save_folder.vi"("Day folder"=w1069, "Measuring number"=w1061, "Measuring folder"="x-U-Scan" ("Subfolder"), "error in"=w1064) -> ("Save Folder"=w1068:string, "Error Out"=w1067:errorcluster)  [unwired: 5 in]
                        n969 = local write "Save folder"(w1068) -> ()
                        n970 = Multiply(x=w1060, y=w1059) -> (x*y=w1062:i32)
                        n971 = local read "Gemittelte Bilder speichern"() -> (w1072:bool)
                        n972 = case shown="True" w1071 {
                          tunnel: w1067 -> [w1074 w1076]
                          tunnel: [w1074 w1075] -> w1066
                          frame #0 {
                          }
                          frame #1 {
                            n973 = local read "Save folder"() -> (w1079:string)
                            n974 = Concatenate Strings(w1079, "\\Einzelbilder" ("Subfolder")) -> (w1077:string)
                            n975 = String To Path(string=w1077) -> (path=w1080:path)
                            n976 = call <vilib>:"Check if File or Folder Exists.vi"("error in (no error)"=w1076, "path"=w1080) -> ("error out"=w1075:errorcluster, "file or folder exists?"=w1081:bool, "dup path"=w1082:path)  [unwired: 7 in]
                            n977 = case shown="False" w1081 {
                              tunnel: w1082 -> [w1083 _]
                              frame #0 {
                                n978 = Create Folder(path (use dialog)=w1083) -> ()  [unwired: 2 in, 3 out]
                              }
                              frame #1 {
                              }
                            }
                          }
                        }
                        n979 = local read "Kamera"() -> (w1073:bool)
                        n980 = local write "# Messschritte"(w1062) -> ()
                        n981 = case shown="True" w1072 {
                          tunnel: w1066 -> [w1084 w1086]
                          tunnel: [w1084 w1085] -> w1065
                          frame #0 {
                          }
                          frame #1 {
                            n982 = local read "Save folder"() -> (w1090:string)
                            n983 = Concatenate Strings(w1090, "\\Gemittelte Bilder" ("Subfolder")) -> (w1092:string)
                            n984 = String To Path(string=w1092) -> (path=w1089:path)
                            n985 = call <vilib>:"Check if File or Folder Exists.vi"("error in (no error)"=w1086, "path"=w1089) -> ("error out"=w1085:errorcluster, "file or folder exists?"=w1088:bool, "dup path"=w1087:path)  [unwired: 7 in]
                            n986 = case shown="False" w1088 {
                              tunnel: w1087 -> [w1093 _]
                              frame #0 {
                                n987 = Create Folder(path (use dialog)=w1093) -> ()  [unwired: 2 in, 3 out]
                              }
                              frame #1 {
                              }
                            }
                          }
                        }
                        n988 = case shown="True" w1073 {
                          tunnel: [w1094 w1096] -> w1063
                          tunnel: w1065 -> [w1094 w1095]
                          frame #0 {
                          }
                          frame #1 {
                            n989 = local read "Ereignis: FrameDone?"() -> (w1097:refnum<event-registration>)
                            n990 = local read "Detektionskamera"() -> (w1098:T4)
                            n991 = call "camera_release_configuration.vi"("error in"=w1095, "Session In"=w1098, "Ereignisregistrierung (Referenz) 2"=w1097) -> ("error out"=w1096:errorcluster)  [unwired: 1 out]
                          }
                        }
                        n992 = local write "Fehler (Ausgang)"(w1063) -> ()
                      }
                    }
                  }
                  frame #1 {
                    n993 = flat-sequence {
                      frame #0 {
                        n994 = local read "x-U-Scan Spannungsstart [V]"() -> (w1105:dbl)
                        n995 = local read "x-U-Scan Rasterschritt [µm]"() -> (w1100:dbl)
                        n996 = local read "x-U-Scan Spannungsschritt [V]"() -> (w1103:dbl)
                        n997 = local read "x-U-Scan Startposition [mm]"() -> (w1104:dbl)
                        n998 = local read "# x-U-Scan Spannungsschritte"() -> (w1107:i32)
                        n999 = local read "# x-U-Scan Rasterschritte"() -> (w1106:i32)
                        n1000 = control-ref of="2D-Intensitätsverteilung (MCP)"() -> (w1102:refnum<vi>)
                        n1001 = Divide(x=w1100, y=1000.0) -> (x/y=w1101:dbl)
                        n1002 = Initialize Array(0.0 ("y"), w1106, w1107) -> (w1111:dbl[][])
                        n1003 = local write "2D-Intensitätsverteilung (MCP)"(w1111) -> ()
                        n1004 = property class="IntGraph (strikt)"(reference=w1102, "XScale.Offset"=w1104, "XScale.Multiplier"=w1101, "YScale.Offset"=w1105, "YScale.Multiplier"=w1103, "XScale.MinorInc"=w1101, "YScale.MinorInc"=w1103, "XScale.NameLbl.Text"="Position [mm]" ("Y-Achse.Namensbeschriftung.Text"), "YScale.NameLbl.Text"="Spannung [V]" ("X-Achse.Namensbeschriftung.Text")) -> (error out=w1110:errorcluster)  [unwired: 1 in, 1 out]
                        n1005 = local write "Fehler (Ausgang)"(w1110) -> ()
                      }
                      frame #1 {
                        n1006 = local write "x-U-Scan läuft"(TRUE ("Messung läuft")) -> ()
                      }
                    }
                  }
                }
              }
            }
          }
          event #6 {
            n1007 = event-data() -> ("NewVal"=w1114:bool)  [unwired: 1 in]
            n1008 = case shown="True" w1114 {
              frame #0 {
              }
              frame #1 {
                n1009 = control-ref of="Shutter time (ms)"() -> (w1150:refnum<vi>)
                n1010 = property class="Ring (strikt)"(reference=w1150) -> ("RingText.Text"=w1132:string)  [unwired: 1 in, 2 out]
                n1011 = local read "# Bilder/Messschritt"() -> (w1128:i32)
                n1012 = local read "Suppressor-Spannung [V]"() -> (w1115:dbl)
                n1013 = local read "P-Schirm-Spannung [V]"() -> (w1120:dbl)
                n1014 = local read "MCP-Spannung [V]"() -> (w1119:dbl)
                n1015 = local read "Leistung (iK) [mW]"() -> (w1118:dbl)
                n1016 = local read "Tip-Spannung [V]"() -> (w1116:dbl)
                n1017 = local read "Polarisation [°]"() -> (w1123:dbl)
                n1018 = local read "Messlogbuch"() -> (w1125:path)
                n1019 = Decimal String To Number(string=w1132) -> (number=w1127:i32)  [unwired: 2 in, 1 out]
                n1020 = local read "Proben-ID"() -> (w1124:string)
                n1021 = Multiply(x=w1128, y=w1127) -> (x*y=w1126:i32)
                n1022 = Concatenate Strings(w1132, "ms_" ("String")) -> (w1131:string)
                n1023 = local read "Sequenz Ordner"() -> (w1148:string)
                n1024 = local read "ROI"() -> (w1121:i32[])
                n1025 = local read "Day folder"() -> (w1149:string)
                n1026 = call "stage_get_current_xyz.vi"() -> ("Aktuelle xyz-Position OUT [mm]"=w1129:dbl[])  [unwired: 3 in, 1 out]
                n1027 = call "create_measure_log_entry.vi"("Messlogbuch-Pfad"=w1125, "Probe"=w1124, "Polarisation [°]"=w1123, "Messart"="Referenzbilder", "ROI"=w1121, "Messungen/Messschritt"=w1128, "Maximalleistung (iK) [mW]"=w1118, "Tip-Spannung [V]"=w1116, "Suppressor-Spannung [V]"=w1115, "Zeit/Messschritt [ms]"=w1127, "MCP-Spannung [V]"=w1119, "Zeit/Messung [ms]"=w1126, "Phosphorschirm-Spannung [V]"=w1120, "xyz [mm]"=w1129) -> ("Messung Nr."=w1117:i32)  [unwired: 4 in, 1 out]
                n1028 = call "create_save_folder.vi"("Day folder"=w1149, "Measuring number"=w1117, "Measuring folder"=w1148) -> ("Save Folder"=w1135:string, "Error Out"=w1146:errorcluster)  [unwired: 6 in]
                n1029 = local write "Save folder"(w1135) -> ()
                n1030 = local read "Kamera"() -> (w1147:bool)
                n1031 = case shown="True" w1147 {
                  tunnel: [w1152 w1155] -> w1138
                  tunnel: w1146 -> [w1152 w1154]
                  tunnel: [w1151 w1153] -> w1137
                  frame #0 {
                    n1032 = local read "Detektionskamera"() -> (w1151:T4)
                  }
                  frame #1 {
                    n1033 = local read "Ereignis: FrameDone?"() -> (w1156:refnum<event-registration>)
                    n1034 = local read "Detektionskamera"() -> (w1157:T4)
                    n1035 = call "camera_release_configuration.vi"("error in"=w1154, "Session In"=w1157, "Ereignisregistrierung (Referenz) 2"=w1156) -> ("error out"=w1155:errorcluster, "Session Out"=w1153:T4)
                  }
                }
                n1036 = local read "# Bilder/Messschritt"() -> (w1144:i32)
                n1037 = call "camera_acquisition_sequence.vi"("Session In"=w1137, "Desired image number"=w1144, "error in"=w1138) -> ("Session Out"=w1136:T4, "Image Array"=w1145:T3[], "error out"=w1143:errorcluster)  [unwired: 1 in]
                n1038 = local read "Buffer Interval"() -> (w1141:u32)
                n1039 = call "save images.vi"("Save Folder"=w1135, "File name prefix"=w1131, "Array"=w1145, "error out 2"=w1143, "Bilder/Messschritt"=w1144) -> ("error out"=w1140:errorcluster)
                n1040 = call "camera_create_configuration.vi"("error in"=w1140, "BufferInterval"=w1141, "Session Out 2"=w1136) -> ("Fehler (Ausgang)"=w1134:errorcluster, "Session Out"=w1139:T4, "Ereignisregistrierung (Referenz)"=w1142:refnum<event-registration>)
                n1041 = local write "Ereignis: FrameDone?"(w1142) -> ()
                n1042 = local write "Detektionskamera"(w1139) -> ()
                n1043 = local write "Fehler (Ausgang)"(w1134) -> ()
                n1044 = Unbundle By Name(w1134) -> ("status"=w1130:bool)
                n1045 = local write "Sequenzaufnahme ON"(w1130) -> ()
              }
            }
          }
        }
        n1046 = local read "Fehler (Ausgang)"() -> (w442:errorcluster)
        n1047 = local read "Programm beenden"() -> (w440:bool)
        n1048 = Unbundle By Name(w442) -> ("status"=w441:bool)
        n1049 = Or(x=w441, y=w440) -> (x .or. y?=w438:bool)
        "Scanschleifenzähler" <- w437
      }
    }
    frame #2 {
      n1050 = flat-sequence {
        frame #0 {
          n1051 = local read "Kamera"() -> (w1218:bool)
          n1052 = case shown="True" w1218 {
            frame #0 {
            }
            frame #1 {
              n1053 = local read "Detektionskamera"() -> (w1220:T4)
              n1054 = local read "Image Memory"() -> (w1222:T3)
              n1055 = call "camera_release configuration_stop.vi"("Image Memory"=w1222, "Detektionskamera"=w1220) -> ("error out"=w1219:errorcluster, "status"=w1221:bool)
              n1056 = local write "Kamera"(w1221) -> ()
              n1057 = local write "Fehler (Ausgang)"(w1219) -> ()
            }
          }
        }
        frame #1 {
          # "Wegen Abstürzen des Programms wird dieser Teil verhindert\nAchtung: IMMER manuell Netzteile auf 0V setzen oder HV-\nSteuerung von Hand ausmachen"
          n1058 = local read "HV-Steuerung"() -> (w1225:bool)
          n1059 = And(x=w1225, y=FALSE) -> (x .and. y?=w1223:bool)
          n1060 = case shown="True" w1223 {
            frame #0 {
            }
            frame #1 {
              n1061 = call "HV_power_supply_set_voltage.vi"("Desired output voltage in V (HV power supply)"=0.0, "Channel of HV power supply"=refnum<k21> "Dev0/Ao1") -> ("error out"=w1226:errorcluster)  [unwired: 8 in]
              n1062 = call "HV_power_supply_set_voltage.vi"("Desired output voltage in V (HV power supply)"=0.0, "Channel of HV power supply"=refnum<k21> "Dev0/Ao0") -> ("error out"=w1227:errorcluster)  [unwired: 8 in]
              n1063 = local write "Fehler (Ausgang)"(w1226) -> ()
              n1064 = local write "Fehler (Ausgang)"(w1227) -> ()
            }
          }
        }
        frame #2 {
          n1065 = local read "Wellenplatte"() -> (w1232:bool)
          n1066 = case shown="True" w1232 {
            frame #0 {
            }
            frame #1 {
              n1067 = local read "Wellenplatte [°]"() -> (w1233:refnum<k7>)
              n1068 = invoke class="MG17Motor" method="StopCtrl"(reference=w1233) -> ()  [unwired: 2 in, 3 out]
            }
          }
        }
        frame #3 {
          w1234 = FALSE ("Bühne bereit")
          w1235 = 0.0 ("Suppressor-Spannung [V]")
          n1069 = local write "Bühne"(w1234) -> ()
          n1070 = local write "Tip-Spannung [V]"(w1235) -> ()
          n1071 = local write "Suppressor-Spannung [V]"(w1235) -> ()
          n1072 = local write "Wellenplatte"(w1234) -> ()
          n1073 = local write "Spannungsscan läuft"(w1234) -> ()
          n1074 = local write "HV-Steuerung"(w1234) -> ()
          n1075 = local write "x-U-Scan läuft"(w1234) -> ()
          n1076 = local write "Waveplate ON/OFF"(w1234) -> ()
          n1077 = local write "x-U-Scan ON/OFF"(w1234) -> ()
          n1078 = local write "Kamera ON/OFF"(w1234) -> ()
        }
      }
    }
  }
